vi "Main Traction Receipe Run.vi"(8 "error in (no error)":errorcluster, 11 "main ref":T1) -> (0 "error out":errorcluster)   [LabVIEW 2025]
uses:
  Traction Receipe Enum.ctl
  v06/controls/LAB-IQ UI Data.ctl
  Temperature/Temperature enum.ctl
  <vilib>/Utility/error.llb/Trim Whitespace One-Sided.vi
panel:
  out "error out 3":errorcluster
  out "error out 2":errorcluster
  in  "Enum - Menu":T2
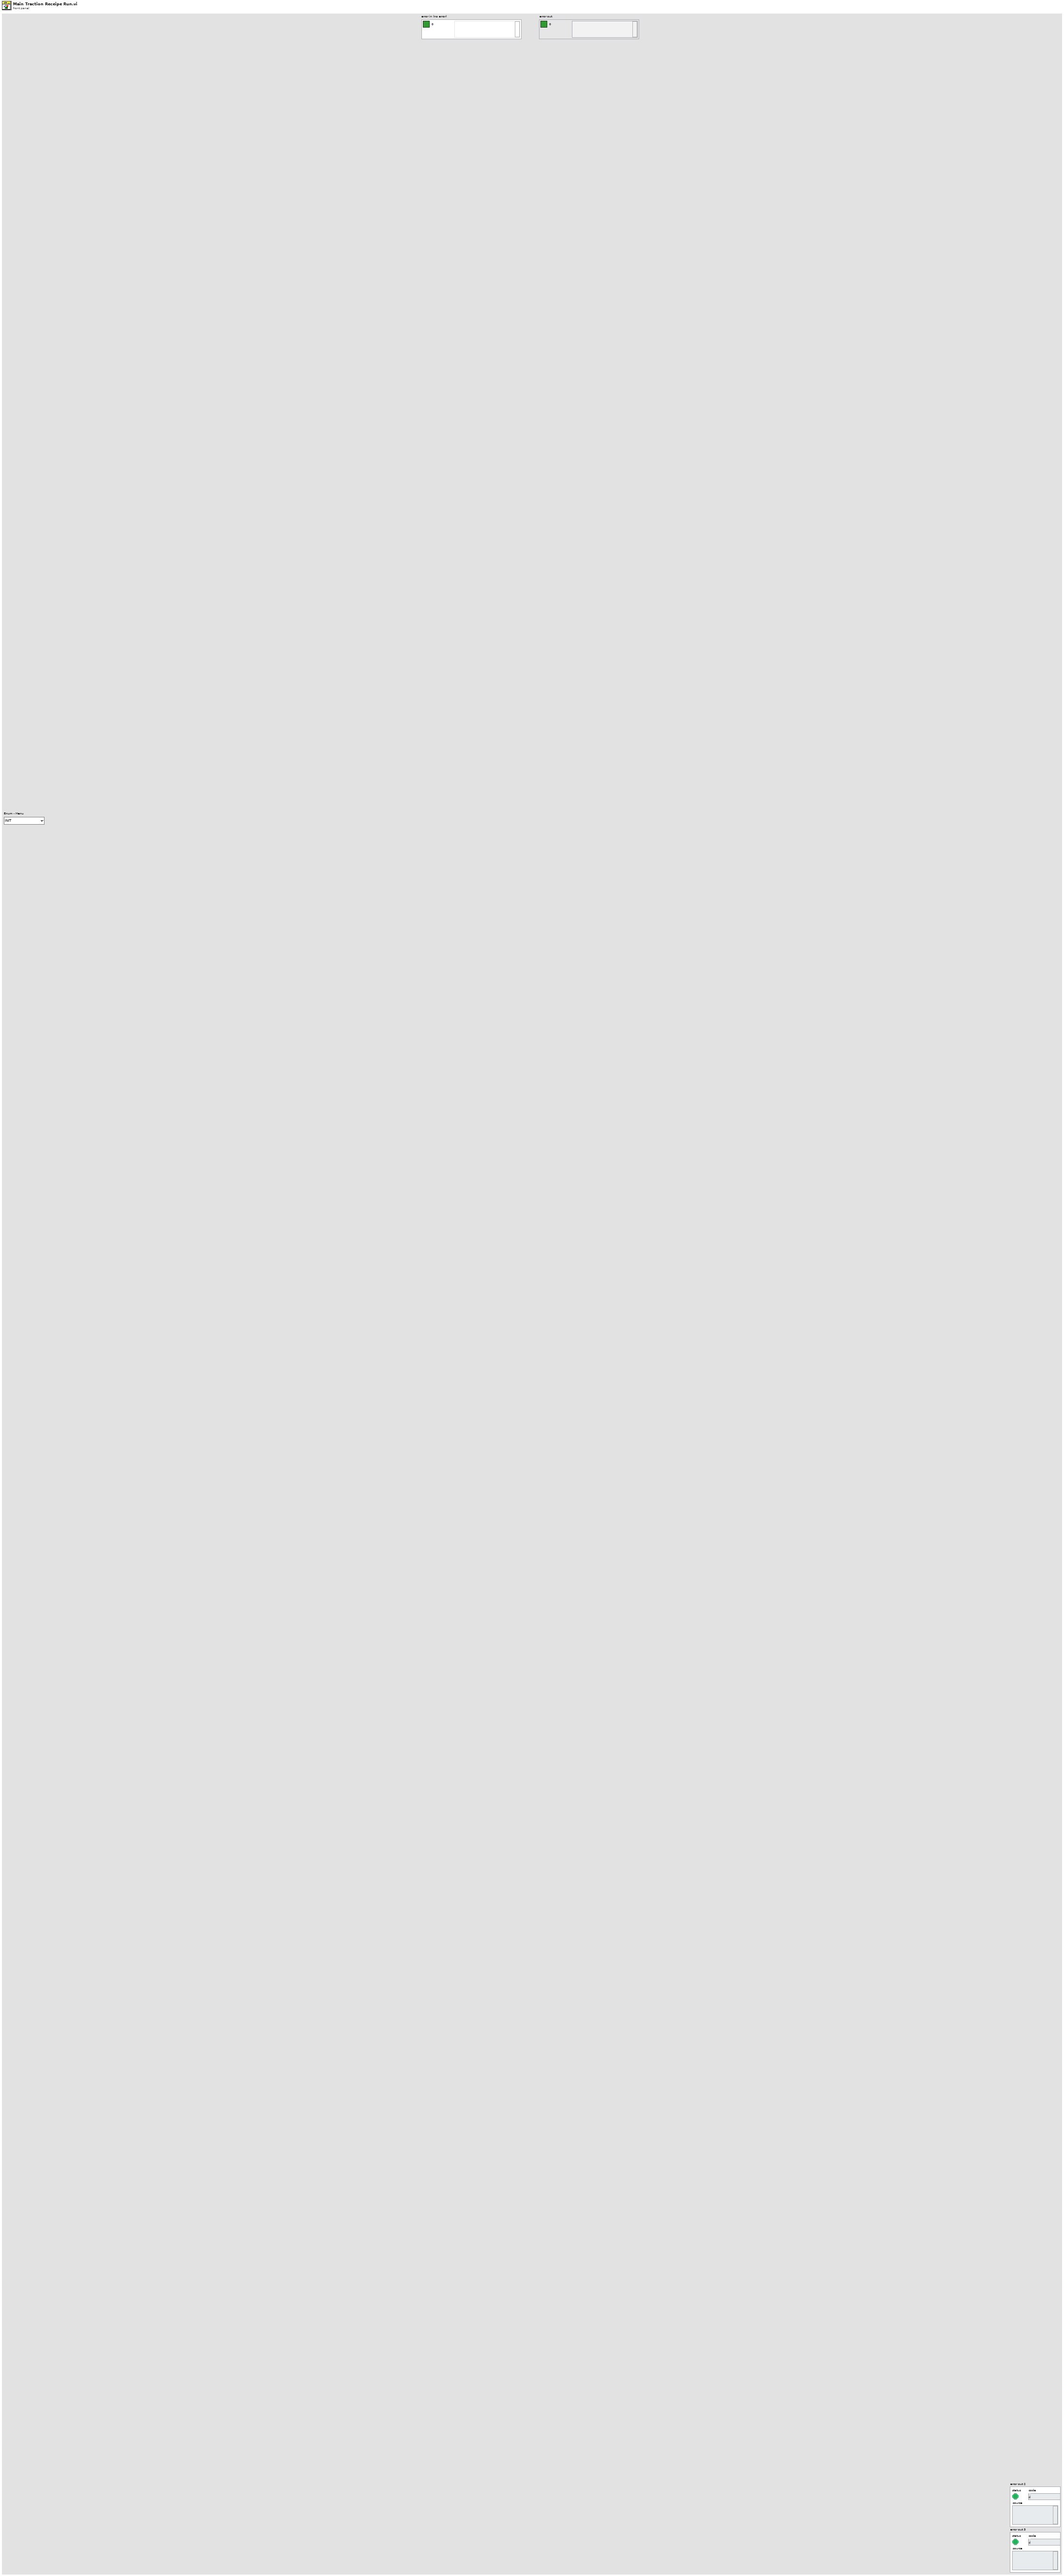
[diagram p1: front panel]
types:
  T1 = typedef "LAB-IQ UI Data.ctl" = cluster{"Main Home Screen":cluster{"GUI":refnum<vi>, "Platform Settings":refnum<vi>, "Configure":refnum<vi>, "Home":refnum<vi>, "EXIT":refnum<vi>, "service 2":refnum<vi>, "MainPage":refnum<vi>, "Analysis":refnum<vi>}, "Platform Settings":cluster{"mm/s  Surge":refnum<vi>, "Drive Error":refnum<vi>, "Disable Axis Jog Soft Limits":refnum<vi>, "mm/s  Sway":refnum<vi>, "Sway and Surge COM Status":refnum<vi>, "Heave COM Status":refnum<vi>, "Enable Platform":refnum<vi>, "Surge Forward Main":refnum<vi>, "Sway Right Main":refnum<vi>, "Sway Left Main":refnum<vi>, "Heave Down Main":refnum<vi>, "Heave Up main":refnum<vi>, "mm/s Heave":refnum<vi>, "mm/sec":refnum<vi>, "mm":refnum<vi>, "Surge Backward Main":refnum<vi>}, "Analysis Screen":cluster{"Analysis Home":refnum<vi>, "Surface Analysis":refnum<vi>, "Imaging":refnum<vi>, "Image Analysis":refnum<vi>, "Post Analysis":refnum<vi>}, "Config Screen":cluster{"Select Load Head":refnum<vi>, "Notes :":refnum<vi>, "FILE":refnum<vi>, "Sample ID :":refnum<vi>, "Operator ID :":refnum<vi>, "Operator Name :":refnum<vi>, "Auto":refnum<vi>}, "Motion Module":cluster{"zNL":refnum<vi>, "NL disp":refnum<vi>, "Rotary Tab":refnum<vi>, "Motion Direction:  3":refnum<vi>, "E.Velocity 2":refnum<vi>, "e.v/ssr 2":refnum<vi>, "Enter Fixed E.Velocity 2":refnum<vi>, "Enter Final SRR 2":refnum<vi>, "Enter initial SRR 2":refnum<vi>, "Enter Fixed SRR 2":refnum<vi>, "Enter the Final E.Velocity (m/s) 2":refnum<vi>, "Enter initial E.Velocity (m/s) 2":refnum<vi>, "Final Speed (RPM) 3":refnum<vi>, "Initial Speed (RPM) 2":refnum<vi>, "Enter the Final Velocity (m/s) 3":refnum<vi>, "Enter initial Velocity (m/s)  3":refnum<vi>, "Ramp Up 2":refnum<vi>, "TEST SELECTION":refnum<vi>, "SPEED SELECTION : ":refnum<vi>, "Angular Oscillation Set":refnum<vi>, "Traction":refnum<vi>, "Step Speed":refnum<vi>, "StepTable For Load-Speed":refnum<vi>, "StepTable For Speed":refnum<vi>, "Surge Forward MM":refnum<vi>, "Surge Backward MM":refnum<vi>, "M3 Image":refnum<vi>, "String 39":refnum<vi>, "Sway Left MM":refnum<vi>, "Sway Right MM":refnum<vi>, "Disable Axis Jog Soft Limits":refnum<vi>, "mm":refnum<vi>, "Heave Down MM":refnum<vi>, "Heave Up MM":refnum<vi>, "Wear Track Diameter (mm)":refnum<vi>, "Set WTD":refnum<vi>, "HomeScratch":refnum<vi>, "HomeRot":refnum<vi>, "PlaceModule":refnum<vi>, "Enter the Angle (Deg)":refnum<vi>, "Enter the Frequency (Hz)":refnum<vi>, "Motion Mode:":refnum<vi>, "LR Sway":refnum<vi>, "Rot Hor":refnum<vi>, "Scratch":refnum<vi>, "LR Cam":refnum<vi>, "MMBack":refnum<vi>, "MMNext":refnum<vi>, "Rot Ver":refnum<vi>, "Rotary Module Selection":refnum<vi>, "calculate rotary":refnum<vi>, "SPEED SELECTION : rotary":refnum<vi>, "Import 2":refnum<vi>, "Save 2":refnum<vi>, "File Path :  2":refnum<vi>, "String 45":refnum<vi>, "StepTable For Speed 3":refnum<vi>, "Enter the Speed(mm/sec)":refnum<vi>, "Enter the Speed(RPM)":refnum<vi>, "Enter Scratch Speed (mm/s):":refnum<vi>, "SwaySpeed Set":refnum<vi>, "Scartch Offset":refnum<vi>, "Motion type:":refnum<vi>, "HomeScratch 2":refnum<vi>, "Enter Scratch length (mm):":refnum<vi>, "Wear Track Diameter":refnum<vi>, "Rotary Speed Exced":refnum<vi>, "Scratch Mode":refnum<vi>, "No of Scratch":refnum<vi>}, "Environmental control":cluster{"Humidity  Status  3":refnum<vi>, "Low Temp  Status  2":refnum<vi>, "TK4 status 2":refnum<vi>, "Stage Temperature":refnum<vi>, "Sample Temperature":refnum<vi>, "Humidity (Amb)":refnum<vi>, "Clear List":refnum<vi>, "Add to list":refnum<vi>, "Wear":refnum<vi>, "Vibration":refnum<vi>, "Humidity (Chamber)":refnum<vi>, "Temperature (Chamber)":refnum<vi>, "ECR ":refnum<vi>, "Temperature (Amb)":refnum<vi>, "Microphone":refnum<vi>, "Acoustic Emission 3":refnum<vi>, "SNext":refnum<vi>, "APBack":refnum<vi>, "Enter the Temperature (°C):":refnum<vi>, "Enter the Stage \nTemperature (°C):":refnum<vi>, "Enter the Humidity (%Rh):":refnum<vi>, "Low Temp":refnum<vi>, "High Temp":refnum<vi>, "Humidity":refnum<vi>, "Sensors Picked":refnum<vi>}, "About Screen":cluster{"Password":refnum<vi>, "Home Service":refnum<vi>, "Advanced Setting":refnum<vi>, "About Tab":refnum<vi>, "ECR Port:":refnum<vi>, "Ramp Port:":refnum<vi>, "Installation/Replacement completed":refnum<vi>, "Loahead":refnum<vi>, "Heave and Surge COM Port:":refnum<vi>, "Sway COM Port:":refnum<vi>, "Temp Modbus:":refnum<vi>, "Humidity Port:":refnum<vi>, "Edit Gain Constants":refnum<vi>, "Save Gain Constants":refnum<vi>}, "Main Screen":cluster{"Main Screen Tab":refnum<vi>, "Angle and Frequency":refnum<vi>, "Stroke (mm)":refnum<vi>, "Angle (Deg)":refnum<vi>, "Main Speed Tab":refnum<vi>, "MTM MOTOR DISPLAY":refnum<vi>, "Disc Speed (m/sec)":refnum<vi>, "Ball Speed (m/sec)":refnum<vi>, "Disc Speed (RPM)":refnum<vi>, "Ball Speed (RPM)":refnum<vi>, "SPEED TAB":refnum<vi>, "Speed (m/sec)":refnum<vi>, "Set Speed (m/sec)":refnum<vi>, "Speed (RPM)":refnum<vi>, "Set Speed":refnum<vi>, "Time Tab":refnum<vi>, "Time ( HH:MM:SS ) 2":refnum<vi>, "Test Duration":refnum<vi>, "Test Duration 4":refnum<vi>, "TEST CYCLE":refnum<vi>, "TOTAL CYCLES":refnum<vi>, "Set Load (N)":refnum<vi>, "Temp Tabs":refnum<vi>, "Heater":refnum<vi>, "TK4 status":refnum<vi>, "ChamberTemp":refnum<vi>, "SetTmp":refnum<vi>, "Controller  Status":refnum<vi>, "ChamberTemp 2":refnum<vi>, "SetTmp 2":refnum<vi>, "Controller  Status 2":refnum<vi>, "ChamberTemp 3":refnum<vi>, "SetTmp 3":refnum<vi>, "Cooling":refnum<vi>, "Load Communication":refnum<vi>, "Ambient \nTemperature":refnum<vi>, "HumCOMStatus":refnum<vi>, "Ambient\n Humidity":refnum<vi>, "Freq (Hz)":refnum<vi>, "Load En":refnum<vi>, "NLt":refnum<vi>, "zNL 2":refnum<vi>, "Humidity On":refnum<vi>, "humidity disp":refnum<vi>, "Set Humidity":refnum<vi>, "NL disp 2":refnum<vi>, "Humidity On 2":refnum<vi>, "humidity disp 2":refnum<vi>, "Set Humidity 2":refnum<vi>, "NL disp 3":refnum<vi>, "AppLoadSeq scratch":refnum<vi>, "Stop Scratch":refnum<vi>, "ClrLog":refnum<vi>, "Trip Log":refnum<vi>, "STOP":refnum<vi>, "Start Test":refnum<vi>, "Test status":refnum<vi>, "AR Led":refnum<vi>, "Data":refnum<vi>, "Health":refnum<vi>, "Sway COM Status":refnum<vi>, "Heave COM Status":refnum<vi>, "Grp Tab":refnum<vi>, "Sub Graph":refnum<vi>, "SD (mm)":refnum<vi>, "Siliding distance Reset Graph":refnum<vi>, "SDGp":refnum<vi>, "Humidity Reset Graph":refnum<vi>, "HumrGp":refnum<vi>, "Acoustic Emission (mV)":refnum<vi>, "Aqucostic Reset Graph":refnum<vi>, "gACQUOS":refnum<vi>, "ECR RESET":refnum<vi>, "ECR":refnum<vi>, "Temperature Reset":refnum<vi>, "Acoustic Emission (mV) 2":refnum<vi>, "Aqucostic Reset Graph 2":refnum<vi>, "gACQUOS 2":refnum<vi>, "ECR RESET 2":refnum<vi>, "ECR 2":refnum<vi>, "Temperature Reset 2":refnum<vi>, "Temperature (deg c)":refnum<vi>, "Speed Reset Graph":refnum<vi>, "Speed Tab":refnum<vi>, "MTM DISC  SPEED":refnum<vi>, "MTM BALL SPEED":refnum<vi>, "speed mm/sec":refnum<vi>, "Hymidity":refnum<vi>, "Humidity Disable trip":refnum<vi>, "CoF Trip  2":refnum<vi>, "Depth Trip":refnum<vi>, "Weart Deapth":refnum<vi>, "Depth Reset Graph":refnum<vi>, "Weart":refnum<vi>, "Depthz":refnum<vi>, "Depth (µm)":refnum<vi>, "WearGp":refnum<vi>, "NL Trip 2":refnum<vi>, "Load pid":refnum<vi>, "Load Disable Trip":refnum<vi>, "Load Reset Graph":refnum<vi>, "NL Display 4":refnum<vi>, "Main Chart 3":refnum<vi>, "BACK":refnum<vi>, "Depth Trip 2":refnum<vi>, "COF TRIP ":refnum<vi>, "Friction Force (N)":refnum<vi>, "FF Reset Graph":refnum<vi>, "FF Disable Trip":refnum<vi>, "FF TRIP":refnum<vi>, "COF Disable Trip":refnum<vi>, "COF Reset Graph":refnum<vi>, "Start Test Temp":refnum<vi>, "zFF":refnum<vi>, "Friction Force (N) Graph":refnum<vi>, "Coefficient of Friction":refnum<vi>, "Scratch Start Test":refnum<vi>, "FF Tab":refnum<vi>, "Cyclic Friction Force (N)":refnum<vi>, "CZ FF":refnum<vi>, "Cyclic Friction Force (N) Graph":refnum<vi>, "Cyclic Coefficient of Friction":refnum<vi>, "Cyclic FF TRIP":refnum<vi>, "Cyclic FF Disable Trip":refnum<vi>, "cyclic COF Disable Trip":refnum<vi>, "cyclic COF TRIP":refnum<vi>, "cyclic COF Reset Graph":refnum<vi>, "Cyclic FF Reset Graph":refnum<vi>, "Test Trip":refnum<vi>, "Multi Scratch Pass":refnum<vi>, "Scratch Start Recording":refnum<vi>, "Coefficient of Friction 2":refnum<vi>, "Acoustic Emission":refnum<vi>, "Friction Force (N) 2":refnum<vi>, "Depth (Microns)":refnum<vi>, "Normal Load ( N )":refnum<vi>}, "Loading":cluster{"Indentation":refnum<vi>, "Reference Sample":refnum<vi>, "Load Cell Communication Slide":refnum<vi>, "com 3":refnum<vi>, "com":refnum<vi>, "DecaForce COM Status":refnum<vi>, "Update":refnum<vi>, "Clear 3":refnum<vi>, "seq":refnum<vi>, "Stribeck table":refnum<vi>, "Stribeck Table  For loading":refnum<vi>, "Loading Mode":refnum<vi>, "Enter the Final Load (N)":refnum<vi>, "Enter the CoF Trip":refnum<vi>, "Enter the Friction Force Trip":refnum<vi>, "Enter the Normal load Trip":refnum<vi>, "Enter the Load  (N)":refnum<vi>, "KiloForce":refnum<vi>, "DecaForce ":refnum<vi>, "MicroForce":refnum<vi>, "LHBack":refnum<vi>, "LHNext":refnum<vi>, "Enter the Loading Rate (N/min)":refnum<vi>, "Message":refnum<vi>, "Warning 2":refnum<vi>, "SSP 0.75":refnum<vi>, "SSP 0.5":refnum<vi>, "SSP 0.3":refnum<vi>, "Warning":refnum<vi>, "gui GIF":refnum<vi>, "Communication is established":refnum<vi>, "AppLoad 4":refnum<vi>, "Multipoint":refnum<vi>, "Load Selection":refnum<vi>}, "PID":cluster{"Ramp":refnum<vi>, "Vertical load (N)":refnum<vi>, "apply load":refnum<vi>, "apply load 2":refnum<vi>, "Enter ByPass Load":refnum<vi>, "Bypass Load":refnum<vi>, "gFF Rot":refnum<vi>}, "Config Parameters":cluster{"Tab Control 3":refnum<vi>, "Tab Control 19":refnum<vi>, "SAMPLES":refnum<vi>, "Re-initilaize":refnum<vi>, "Filter ON/OFF":refnum<vi>, "TracHomeSurgeOffsetCounts 10MM":refnum<vi>, "TracHomeSwayOffsetCounts 10MM":refnum<vi>, "Acoustic Emission:":refnum<vi>, "Apply Filter (FF)":refnum<vi>, "Filter% 2":refnum<vi>, "Apply Filter (Load)":refnum<vi>, "Filter% ":refnum<vi>, "Sway distance (mm)":refnum<vi>, "Surge distance (mm)":refnum<vi>, "DataSavingLoopDelay(ms)":refnum<vi>, "SAVE 2":refnum<vi>, "Enter Distance":refnum<vi>, "Sway Counts:":refnum<vi>, "Distance (mm): 3":refnum<vi>, "Surge Counts:":refnum<vi>, "Distance (mm): 2":refnum<vi>, "Distance (mm):":refnum<vi>, "Heave Counts:":refnum<vi>, "LRMHomeSurgeOffsetCounts":refnum<vi>, "LRMHomeSwayOffsetCounts":refnum<vi>, "TracHomeSurgeOffsetCounts 20MM":refnum<vi>, "TracHomeSwayOffsetCounts 20MM":refnum<vi>, "RotHomeSwayOffsetCounts":refnum<vi>, "RotHomeSurgeOffsetCounts":refnum<vi>, "Heave distance":refnum<vi>, "Zmm":refnum<vi>, "Heave Pulses/mm":refnum<vi>, "Surge Pulses/mm":refnum<vi>, "Sway Pulses/mm":refnum<vi>, "Heave Pitch":refnum<vi>, "Surge Pitch":refnum<vi>, "Sway Pitch":refnum<vi>, "Heave PPR":refnum<vi>, "Surge PPR":refnum<vi>, "Sway PPR":refnum<vi>, "Tab Control 5":refnum<vi>, "Tab Control 14":refnum<vi>, "Tab Control 26":refnum<vi>, "AE":refnum<vi>, "Heave Loop Delay":refnum<vi>, "Heave PID Speed":refnum<vi>, "Surge Jog Speed":refnum<vi>, "Heave Jog Speed":refnum<vi>, "Sway Loop Delay":refnum<vi>, "Sway PID Speed":refnum<vi>, "Sway Jog Speed":refnum<vi>, "DEPTH TRIP VALUE":refnum<vi>, "LOAD TRIP VALUE":refnum<vi>, "DEPTH TRIP   ENABLE":refnum<vi>, "LOAD TRIP  ENABLE":refnum<vi>, "CYCLIC FF TRIP VALUE":refnum<vi>, "FF TRIP VALUE":refnum<vi>, "CYCLIC CoF TRIP VALUE":refnum<vi>, "COF TRIP VALUE":refnum<vi>, "CYCLIC COF TRIP  ENABLE":refnum<vi>, "CYCLIC FF TRIP  ENABLE":refnum<vi>, "FF TRIP  ENABLE":refnum<vi>, "COF TRIP  ENABLE":refnum<vi>, "JOG TRIP LOAD VALUE (N)":refnum<vi>, "Rotary Vertical":refnum<vi>, "Traction":refnum<vi>, "Scratch":refnum<vi>, "LRM CAM":refnum<vi>, "Sway LRM":refnum<vi>, "Rotary Horizontal":refnum<vi>, "SURGE SPEED":refnum<vi>, "SURGE BACKWARD COUNT":refnum<vi>, "SURGE FORWARD COUNT":refnum<vi>, "Start Button":refnum<vi>}, "Loading Com Port":cluster{"ClearAll":refnum<vi>, "Mz(Nm)":refnum<vi>, "My(Nm)":refnum<vi>, "Mx(Nm)":refnum<vi>, "Save Dwell":refnum<vi>, "Acq Delay (ms)":refnum<vi>, "Burst Delay (ms)":refnum<vi>, "model":refnum<vi>, "SN":refnum<vi>, "FFx(N)":refnum<vi>, "Sensor IP":refnum<vi>, "Port":refnum<vi>, "FFy(N)":refnum<vi>, "Load(N)":refnum<vi>, "delete Handle":refnum<vi>, "Create Handle":refnum<vi>, "ft_data":refnum<vi>, "ft_range":refnum<vi>, "ft_data 2":refnum<vi>, "stop 6":refnum<vi>, "running_flag":refnum<vi>, "ft_udp_handle":refnum<vi>, "get-data-return":refnum<vi>, "get-range-return":refnum<vi>, "zero-return":refnum<vi>, "filter-return":refnum<vi>, "initial-return":refnum<vi>, "deleteHandle-result":refnum<vi>, "Load Cell Temp":refnum<vi>, "Load Cell":refnum<vi>, "ZeroAll":refnum<vi>, "FORCE (N)":refnum<vi>, "TORQUE (N-m)":refnum<vi>, "Load Cell Link":refnum<vi>}, "Heave AND Surge":cluster{"SURGE POSE":refnum<vi>, "error out Read":refnum<vi>, "HEAVE POSE":refnum<vi>, "State":refnum<vi>, "Homed":refnum<vi>, "Sequence ID":refnum<vi>, "error out Write":refnum<vi>, "faultCode":refnum<vi>, "Ack ID":refnum<vi>, "SPEED":refnum<vi>, "Distance":refnum<vi>, "Mode Command":refnum<vi>, "Heave and Surge Read":refnum<vi>, "Read Heave Temp":refnum<vi>, "Spare 15":refnum<vi>, "Spare 14":refnum<vi>, "Spare 13":refnum<vi>, "Spare 12":refnum<vi>, "Spare 11":refnum<vi>, "Spare 10":refnum<vi>, "Spare 9":refnum<vi>, "Spare 8":refnum<vi>, "Spare 7":refnum<vi>, "Spare 4":refnum<vi>, "Spare 3":refnum<vi>, "Spare 2":refnum<vi>, "Humidity":refnum<vi>, "Temp":refnum<vi>, "Node Id":refnum<vi>, "Spare 1":refnum<vi>, "SPARE 4":refnum<vi>, "SPARE 3":refnum<vi>, "SPARE 2":refnum<vi>, "SPARE 1":refnum<vi>, "fwMajor":refnum<vi>, "fwMinor":refnum<vi>, "Manual Write":refnum<vi>, "Heave and Surge Write":refnum<vi>, "SPARE 5":refnum<vi>, "Reserved ":refnum<vi>, "SPARE 8":refnum<vi>, "SPARE 6":refnum<vi>, "SPARE 7":refnum<vi>, "SPARE 17":refnum<vi>, "SPARE 16":refnum<vi>, "SPARE 15":refnum<vi>, "SPARE 14":refnum<vi>, "SPARE 13":refnum<vi>, "SPARE 12":refnum<vi>, "SPARE 11":refnum<vi>, "SPARE 10":refnum<vi>, "SPARE 9":refnum<vi>, "System UPTIME":refnum<vi>, "Missed Packets":refnum<vi>, "faultCode Surge Right":refnum<vi>, "faultCode Surge Left":refnum<vi>, "faultCode Heave":refnum<vi>, "UPLINK HEAVE":refnum<vi>, "DOWNLINK HEAVE":refnum<vi>}, "New PID LOGIC":cluster{"Fine Tune Zone":refnum<vi>, "PID SDelay":refnum<vi>, "Max_pos_limit":refnum<vi>, "Min_pos_limit":refnum<vi>, "i_limit":refnum<vi>, "pct_scale":refnum<vi>, "Deadband":refnum<vi>, "Kd":refnum<vi>, "Ki":refnum<vi>, "Kp":refnum<vi>, "Current Position":refnum<vi>, "Set Load":refnum<vi>, "Current Load":refnum<vi>, "Pulse delta":refnum<vi>, "Init Step":refnum<vi>, "Max Step Linit":refnum<vi>, "min_deadband_floor":refnum<vi>, "dynamic_spindle_noise_scalar":refnum<vi>, "min_finetune_floor":refnum<vi>, "filter_alpha":refnum<vi>, "PID":refnum<vi>}, "SWAY ":cluster{"fwMajor":refnum<vi>, "Homed":refnum<vi>, "Rotary POSE":refnum<vi>, "State":refnum<vi>, "SWAY POSE":refnum<vi>, "Ack ID":refnum<vi>, "faultCode":refnum<vi>, "Node Id":refnum<vi>, "fwMinor":refnum<vi>, "Spare 6":refnum<vi>, "Spare 5":refnum<vi>, "Spare 4":refnum<vi>, "Spare 3":refnum<vi>, "Spare 2":refnum<vi>, "Spare 1":refnum<vi>, "Spare 7":refnum<vi>, "SPARE  5":refnum<vi>, "error out Write  SWAY ":refnum<vi>, "error out Read SWAY ":refnum<vi>, "Manual Write SWAY ":refnum<vi>, "SWAY WRITE":refnum<vi>, "SPARE  4":refnum<vi>, "SPARE  3":refnum<vi>, "SPARE 2":refnum<vi>, "SPARE 1":refnum<vi>, "Spare 15":refnum<vi>, "Spare 14":refnum<vi>, "Spare 13":refnum<vi>, "Spare 12":refnum<vi>, "Spare 11":refnum<vi>, "Spare 9":refnum<vi>, "Spare 8":refnum<vi>, "SPEED":refnum<vi>, "Distance":refnum<vi>, "Mode Command":refnum<vi>, "Sequence ID":refnum<vi>, "SWAY READ":refnum<vi>, "Spare 10":refnum<vi>, "Read SWAY Temp":refnum<vi>, "faultCode Sway ":refnum<vi>, "Missed Packets":refnum<vi>, "System UPTIME sway":refnum<vi>, "SPARE 6":refnum<vi>, "SPARE 7":refnum<vi>, "SPARE 9":refnum<vi>, "SPARE 11":refnum<vi>, "SPARE 10":refnum<vi>, "SPARE 8":refnum<vi>, "SPARE 13":refnum<vi>, "SPARE 12":refnum<vi>, "SPARE 17":refnum<vi>, "SPARE 16":refnum<vi>, "SPARE 15":refnum<vi>, "SPARE 14":refnum<vi>, "Reserved":refnum<vi>, "faultCode Rotary":refnum<vi>, "UPLINK SWAY":refnum<vi>, "DOWNLINK SWAY":refnum<vi>}, "Analysis Screen":cluster{"Analysis Home":refnum<vi>, "Refresh 2":refnum<vi>, "MEAN 4":refnum<vi>, "SD 4":refnum<vi>, "VARIANCE 4":refnum<vi>, "MEAN  3":refnum<vi>, "SD  3":refnum<vi>, "VARIANCE  3":refnum<vi>, "MEAN 2":refnum<vi>, "SD  2":refnum<vi>, "VARIANCE 2":refnum<vi>, "MEAN":refnum<vi>, "SD":refnum<vi>, "VARIANCE":refnum<vi>, "File 4 Discription":refnum<vi>, "OPEN 4":refnum<vi>, "File Name 4":refnum<vi>, "OPEN 3":refnum<vi>, "File 3 Discription":refnum<vi>, "File Name 3":refnum<vi>, "Y-AXIS":refnum<vi>, "X-AXIS":refnum<vi>, "XY Graph":refnum<vi>, "File Name 2":refnum<vi>, "File Name 1":refnum<vi>, "OPEN 2":refnum<vi>, "OPEN 1":refnum<vi>, "File 1 Discription ":refnum<vi>, "File 2 Discription":refnum<vi>, "Export":refnum<vi>, "File Format":refnum<vi>}, "Traction":cluster{"faultCode Traction 2":refnum<vi>, "faultCode Traction 1":refnum<vi>, "Missed Packets":refnum<vi>, "System UPTIME Traction":refnum<vi>, "SPARE 17":refnum<vi>, "SPARE 16":refnum<vi>, "SPARE 15":refnum<vi>, "SPARE 14":refnum<vi>, "SPARE 13":refnum<vi>, "SPARE 12":refnum<vi>, "SPARE 11":refnum<vi>, "SPARE 10":refnum<vi>, "SPARE 9":refnum<vi>, "SPARE 8":refnum<vi>, "SPARE 7":refnum<vi>, "SPARE 6":refnum<vi>, "Reserved":refnum<vi>, "SPARE  5":refnum<vi>, "Manual Write TRACTION":refnum<vi>, "TRACTION WRITE":refnum<vi>, "SPARE  4":refnum<vi>, "SPARE  3":refnum<vi>, "SPARE 2":refnum<vi>, "SPARE 1":refnum<vi>, "Spare 7":refnum<vi>, "Spare 6":refnum<vi>, "Spare 5":refnum<vi>, "Spare 4":refnum<vi>, "Spare 2":refnum<vi>, "Spare 1":refnum<vi>, "Node Id":refnum<vi>, "Read TRACTION Temp":refnum<vi>, "fwMinor":refnum<vi>, "fwMajor":refnum<vi>, "faultCode":refnum<vi>, "TRACTION POSE":refnum<vi>, "TRACTION POSE 2":refnum<vi>, "Homed":refnum<vi>, "State":refnum<vi>, "Ack ID":refnum<vi>, "SPEED":refnum<vi>, "Distance":refnum<vi>, "Mode Command":refnum<vi>, "Sequence ID":refnum<vi>, "error out Read TRACTION":refnum<vi>, "error out Write  TRACTION":refnum<vi>, "TRACTION READ":refnum<vi>, "Spare 3":refnum<vi>, "Downlink traction":refnum<vi>, "Uplink Traction":refnum<vi>}, "Traction reciepe":cluster{"SRR Sweep Range (%) Stribeck":refnum<vi>, "Traction Receipe":refnum<vi>, "Total Execution Time":refnum<vi>, "Total Steps":refnum<vi>, "Duration / Step (s)  Stribeck":refnum<vi>, "STRIBECK Fixed SRR List (%)":refnum<vi>, "Duration / Step (s) Traction":refnum<vi>, "SRR Sweep Range (%) traction":refnum<vi>, "Rolling Speed (mm/s)":refnum<vi>, "Temperature Stages (°C)":refnum<vi>, "Ball Load (N)":refnum<vi>, "Lubricant Name":refnum<vi>, "Profile File Name":refnum<vi>, "SET entrainment Velocity":refnum<vi>, "Test Array Size":refnum<vi>, "SRR INDEX [ STRIBECK]":refnum<vi>, "Stribeck Size":refnum<vi>, "SET SRR":refnum<vi>, "ELAPSED TIMER ":refnum<vi>, "BALL SET RPM":refnum<vi>, "DISC SET RPM":refnum<vi>, "SET LOAD":refnum<vi>, "TEMPERATURE READ":refnum<vi>, "SET TEMPERATURE":refnum<vi>, "Traction Size":refnum<vi>, "DISC SPEED (rpm)":refnum<vi>, "BALL SPEED (rpm)":refnum<vi>, "BALL WEAR TRACK":refnum<vi>, "DISC WEARTRACK":refnum<vi>, "SRR INDEX [ TRACTION]":refnum<vi>, "Start Index Type":refnum<vi>, "Enum - Menu":refnum<vi>, "Ball (mm/sec)":refnum<vi>, "Disc (mm/sec)":refnum<vi>, "Traction Receipe Update Details":refnum<vi>}, "Traction Control":cluster{"HomeTraction":refnum<vi>, "Demo Mode Display":refnum<vi>, "Traction Message":refnum<vi>, "Traction Step Update Details":refnum<vi>, "Main Tab sequence for selection":refnum<vi>, "Ramp Tab":refnum<vi>, "e.v/ssr":refnum<vi>, "Enter Fixed E.Velocity":refnum<vi>, "Enter Final SRR":refnum<vi>, "Enter initial SRR":refnum<vi>, "Enter Fixed SRR":refnum<vi>, "Enter the Final E.Velocity (m/s)":refnum<vi>, "Enter initial E.Velocity (m/s)":refnum<vi>, "Ball WTD":refnum<vi>, "E.Velocity":refnum<vi>, "Enter the Final Velocity (m/s)":refnum<vi>, "Enter initial Velocity (m/s)":refnum<vi>, "Ramp Up   Disc":refnum<vi>, "Initial DiscSpeed (RPM)":refnum<vi>, "Final Speed (RPM) Ball":refnum<vi>, "Final Speed (RPM)":refnum<vi>, "Initial Speed (RPM) Ball":refnum<vi>, "Enter the Final Velocity (m/s) Ball":refnum<vi>, "Enter initial Velocity (m/s) Ball":refnum<vi>, "Ramp Up":refnum<vi>, "ExceedBallSpeed step":refnum<vi>, "ExceedDiscSpeed":refnum<vi>, "BallSpeed Exceed Indication":refnum<vi>, "Apply":refnum<vi>, "SPEED SELECTION : MTM":refnum<vi>, "SPEED SELECTION : MTM 2":refnum<vi>, "TEST SELECTION (MTM)":refnum<vi>, "MTM Test Selection":refnum<vi>, "File Path Tab":refnum<vi>, "File Path String":refnum<vi>, "Save":refnum<vi>, "Save  2":refnum<vi>, "Import ":refnum<vi>, "File Path :":refnum<vi>, "Step Sequence Indication Tab":refnum<vi>, "Step Sequence Indication":refnum<vi>, "Calculate Step":refnum<vi>, "StepTable":refnum<vi>, "ExceedDiscSpeed  Cinstant Speed":refnum<vi>, "ExceedBallSpeed Constant":refnum<vi>, "TEST SELECTION (MTM) 2":refnum<vi>, "SPEED SELECTION : MTM 3":refnum<vi>, "MTM Test Selection 2":refnum<vi>, "Enter the Speed (m/sec): ":refnum<vi>, "Enter the Speed (m/sec):  2":refnum<vi>, "Enter the Speed (RPM):":refnum<vi>, "Lower Spped ":refnum<vi>, "Upper":refnum<vi>, "Enter the Speed (RPM):Ball":refnum<vi>, "Disc Motion Direction: ":refnum<vi>, "Ball Motion Direction :":refnum<vi>, "Motion Mode: ":refnum<vi>, "Wear Track Diameter (mm) ":refnum<vi>, "Disc Speed Indicator":refnum<vi>, "ExceedBallSpeed":refnum<vi>}, "Acquostic":cluster{"Last Config Rejected ":refnum<vi>, "rx command count":refnum<vi>, "Current Filter Id":refnum<vi>, "Isolated Gain":refnum<vi>, "DAQ Status":refnum<vi>, "error out":refnum<vi>, "error in (no error)":refnum<vi>, "Uplink Packet":refnum<vi>, "data out":refnum<vi>, "Downlink Packet":refnum<vi>, "Gains":refnum<vi>, "Manual Write Acquostic":refnum<vi>, "Acoustic Graphs":refnum<vi>}, "ABOUT":cluster{"version":refnum<vi>, "Operating System":refnum<vi>, "Version":refnum<vi>, "Workorder":refnum<vi>, "Runtime":refnum<vi>, "Instrument Serial":refnum<vi>, "Firmware Version":refnum<vi>, "Info":refnum<vi>}, "Temperature Port":cluster{"Temperature":refnum<vi>, "error out Temperature":refnum<vi>, "READ TEMPERATURE":refnum<vi>}}
  T2 = typedef "Traction Receipe Enum.ctl" = enum16{"INIT", "START", "TRACTION", "STRIBECK", "MAIN INDEX INCREMENT", "TEMPERATURE SET", "TEMPERATURE REACH", "CHURNING START", "CHURNING STOP", "LOAD", "LOAD REACHED", "SRR SET", "SRR WAIT", "SRR INCREMENT", "SPEED SET", "SPEED WAIT", "SPEED INCREMENT", "UNLOAD", "CLOSE"}
  T3 = typedef "Temperature enum.ctl" = enum16{"Init", "read", "write", "close", "error_init"}
  T4 = enum8{"Enabled", "Disabled", "Disabled and Grayed Out"}
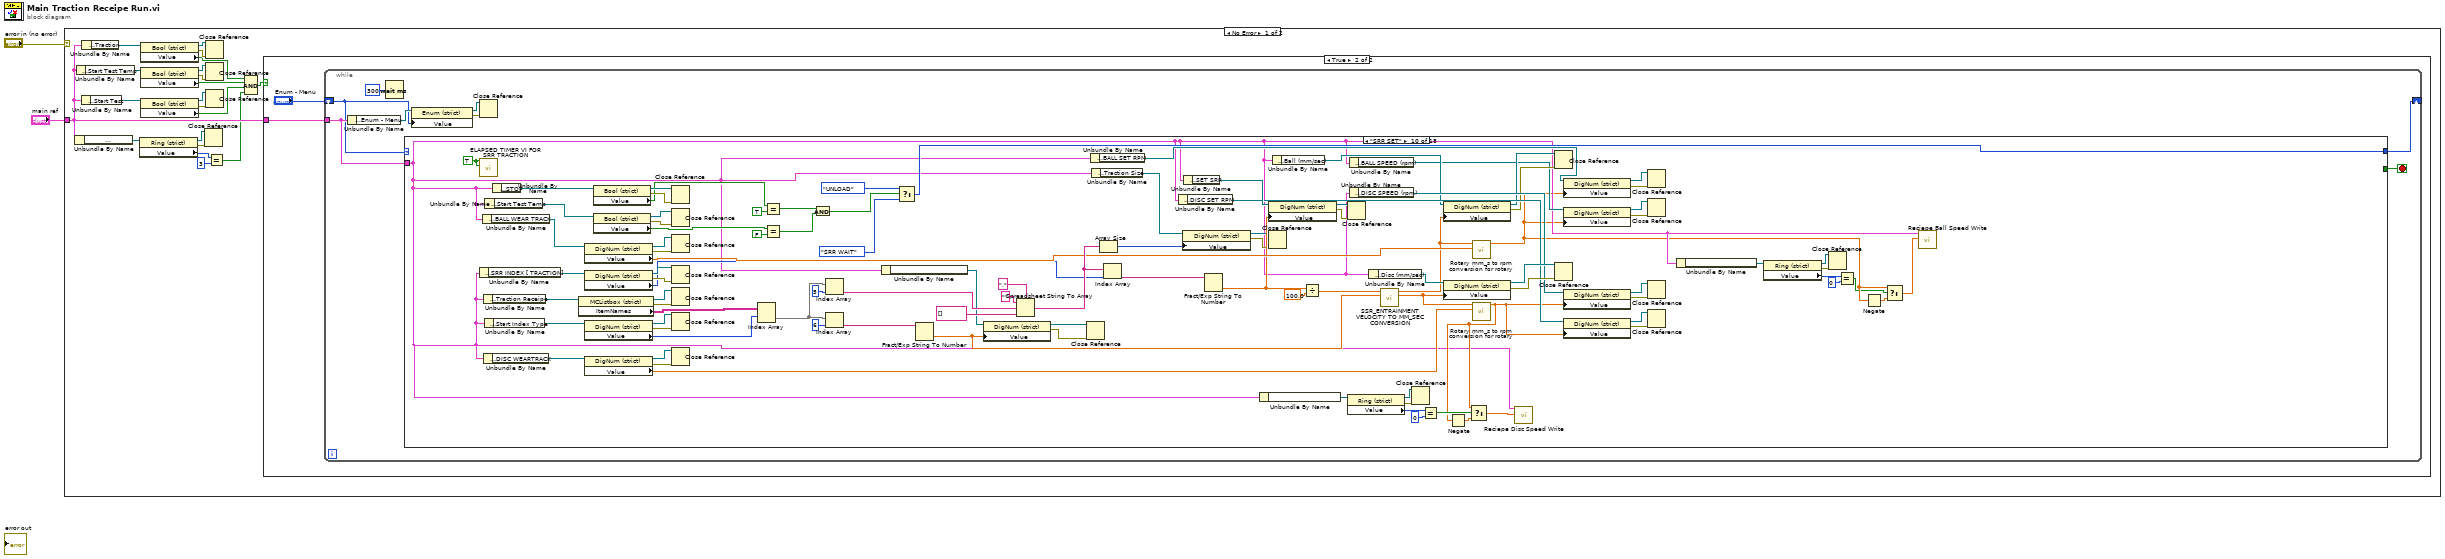
[diagram p0: block diagram]
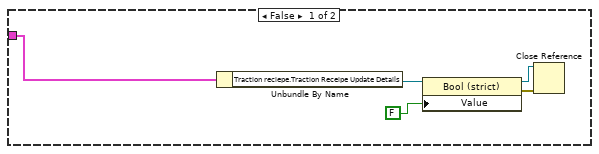
[diagram p2: hidden frame]
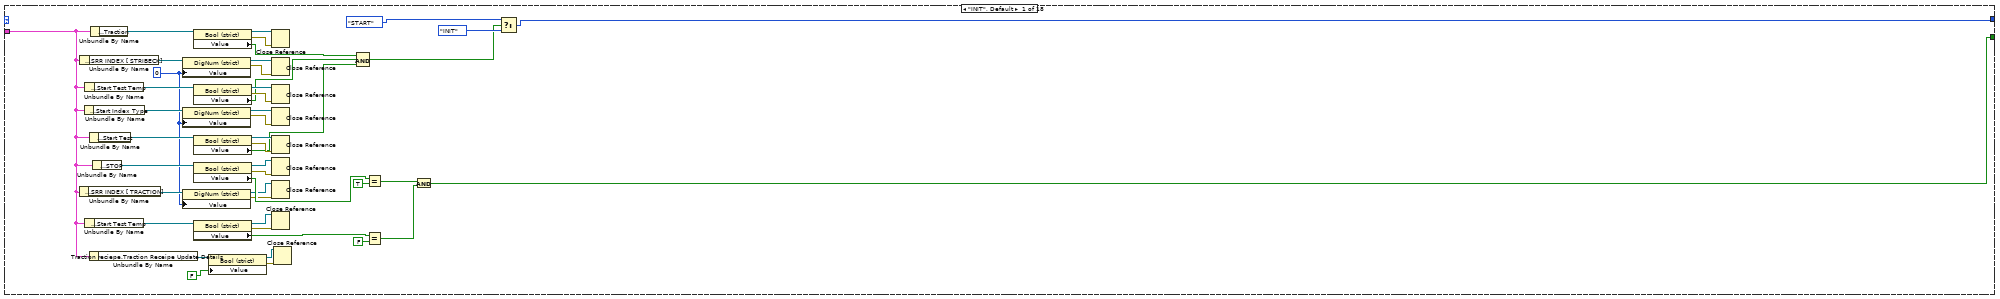
[diagram p3: hidden frame]
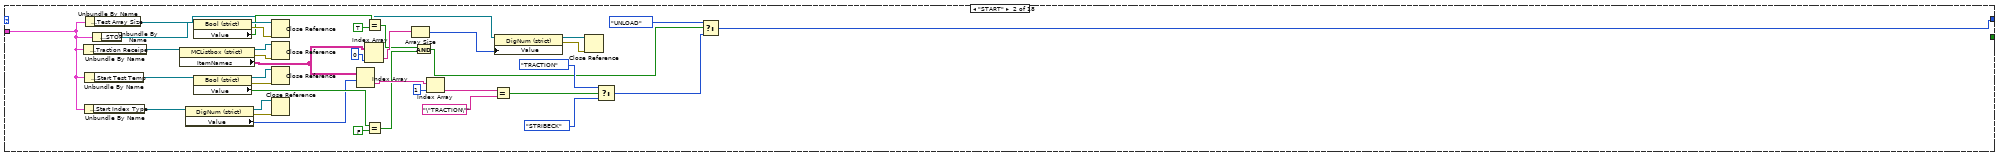
[diagram p4: hidden frame]
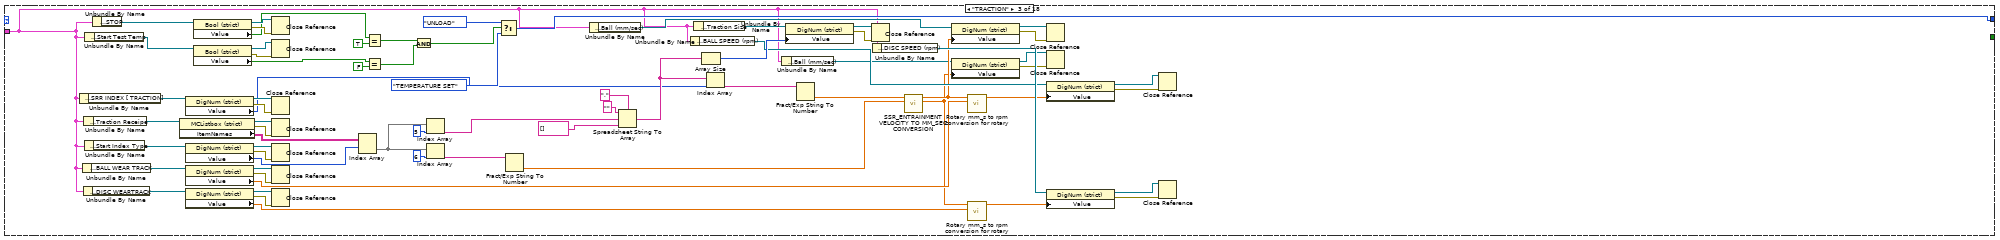
[diagram p5: hidden frame]
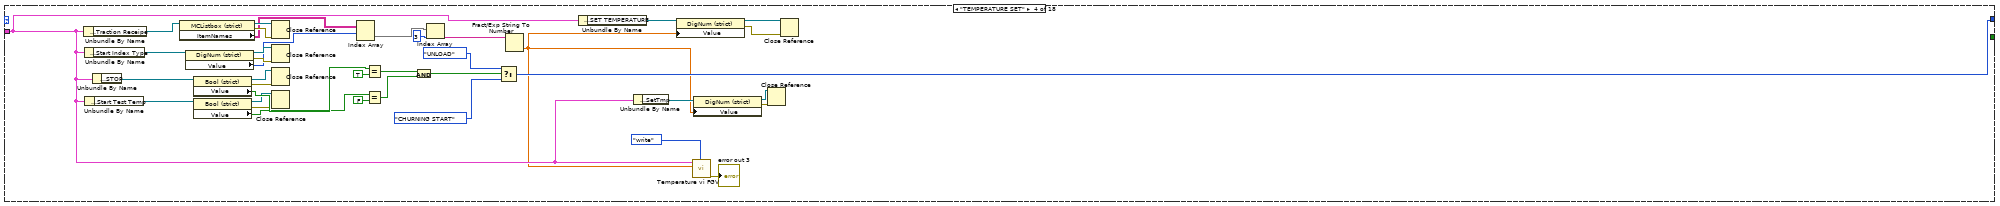
[diagram p6: hidden frame]
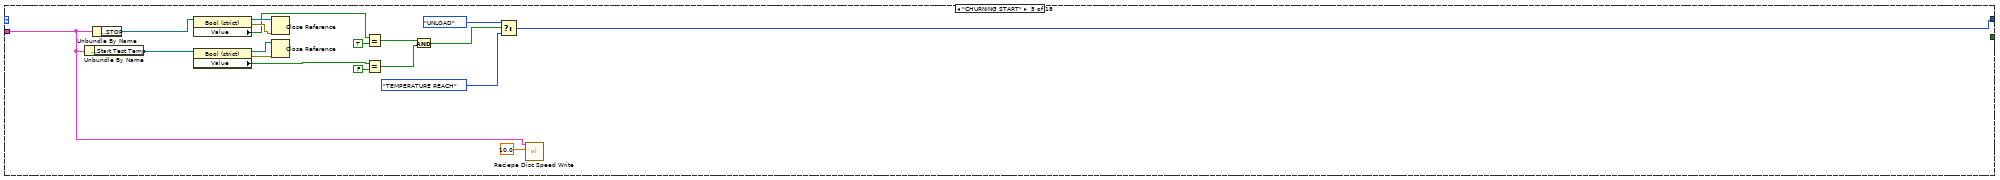
[diagram p7: hidden frame]
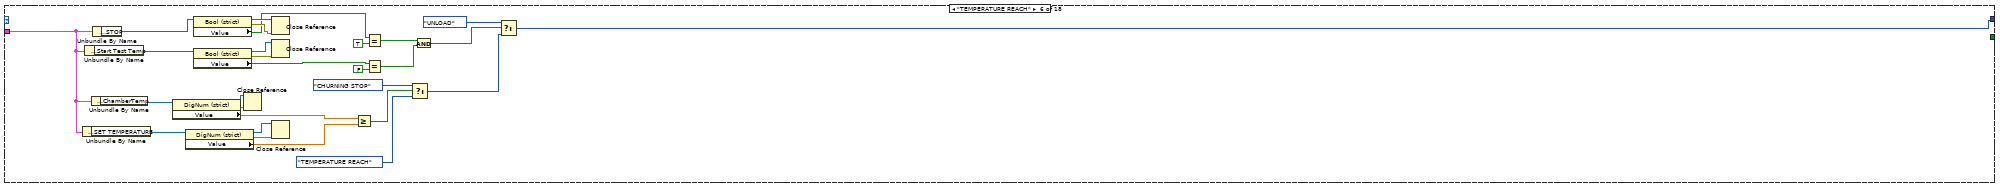
[diagram p8: hidden frame]
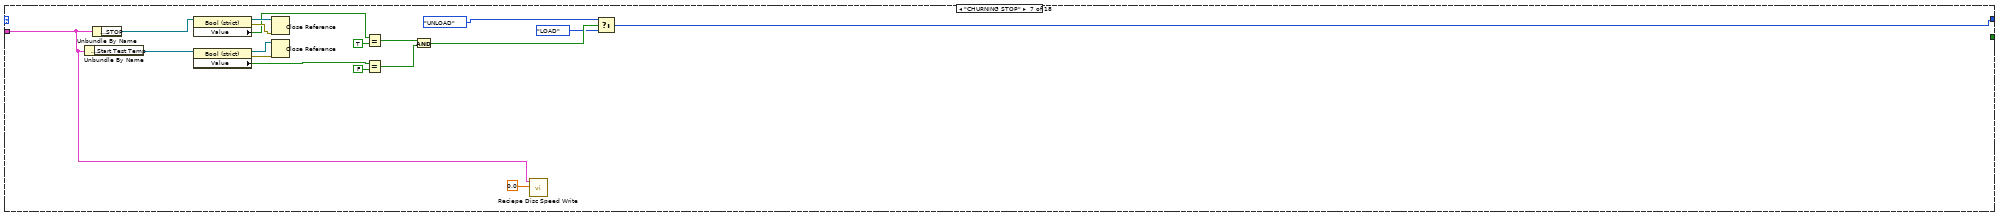
[diagram p9: hidden frame]
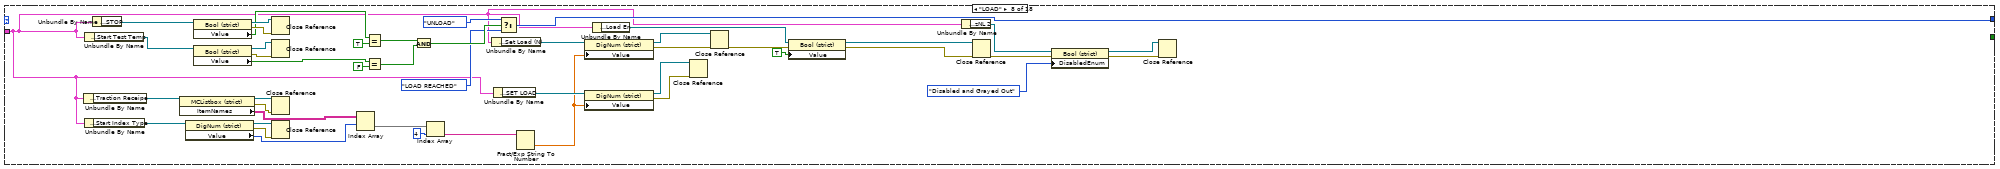
[diagram p10: hidden frame]
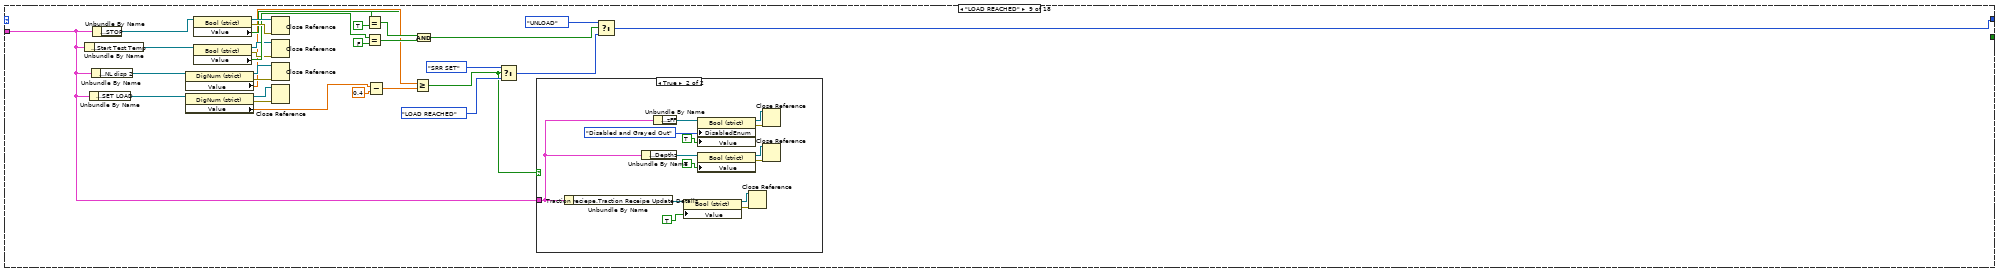
[diagram p11: hidden frame]
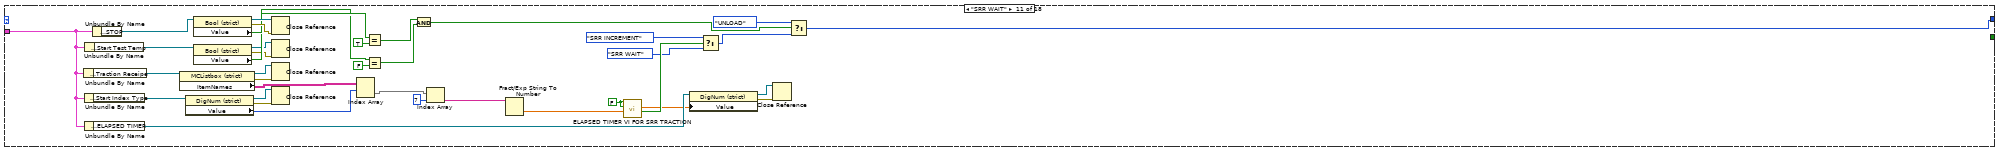
[diagram p13: hidden frame]
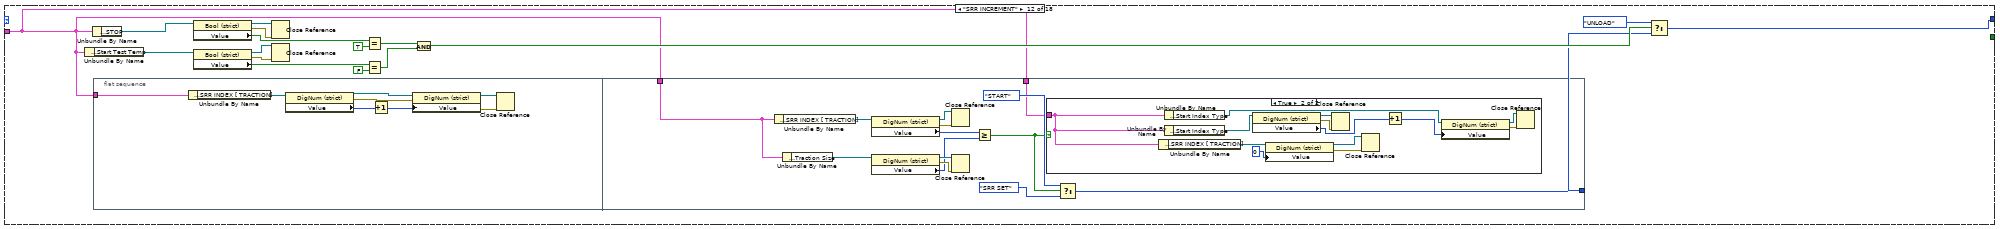
[diagram p14: hidden frame]
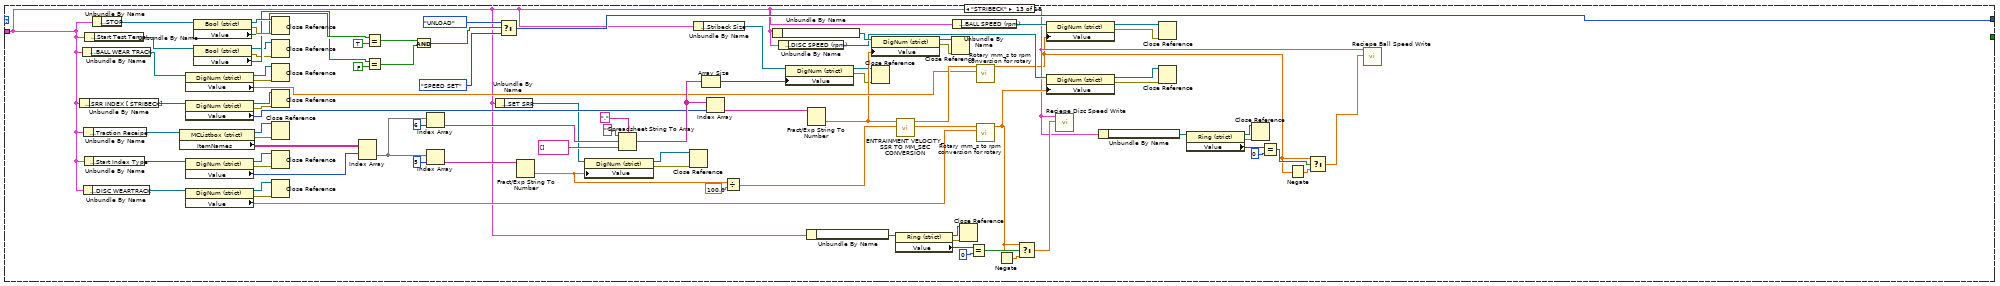
[diagram p16: hidden frame]
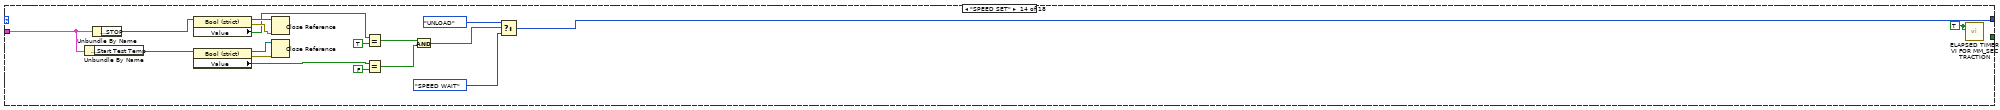
[diagram p17: hidden frame]
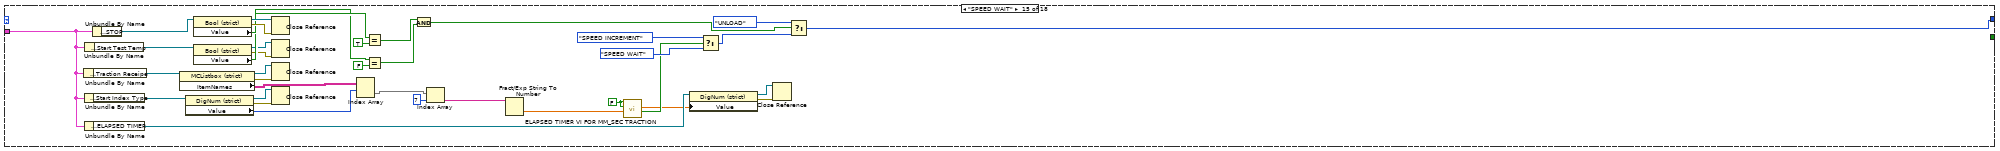
[diagram p18: hidden frame]
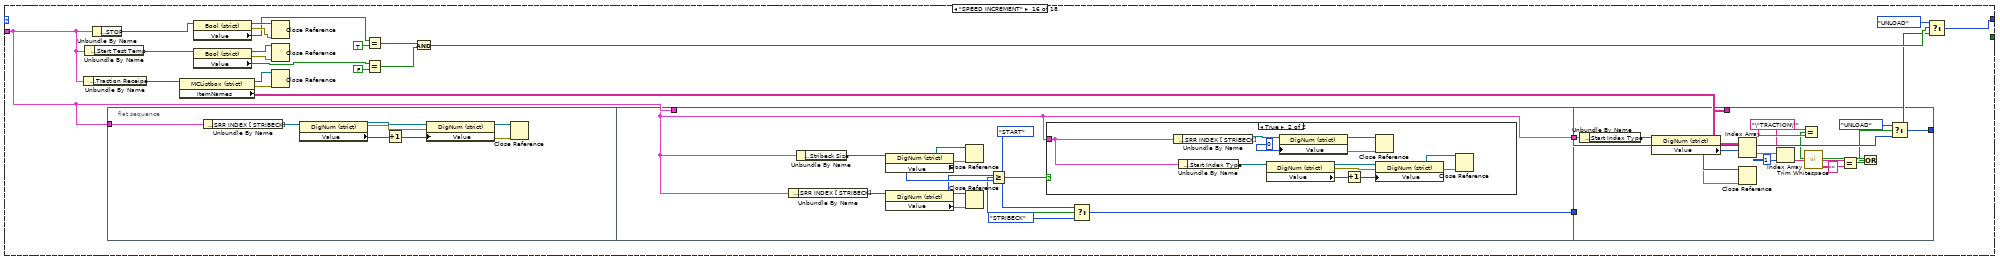
[diagram p19: hidden frame]
diagram:
  n1 = case shown="No Error" "error in (no error)" {
    tunnel: "main ref" -> [w6 _]
    frame No Error {
      n2 = Unbundle By Name(w6) -> ("Traction Control.Motion Mode:"=w8:refnum<vi>)
      n3 = Unbundle By Name(w6) -> ("Main Screen.Start Test Temp"=w21:refnum<vi>)
      n4 = Unbundle By Name(w6) -> ("Main Screen.Start Test"=w18:refnum<vi>)
      n5 = Unbundle By Name(w6) -> ("Motion Module.Traction"=w13:refnum<vi>)
      n6 = property class="Ring (strict)"(reference=w8) -> (reference out=w9:refnum<vi>, error out=w7:errorcluster, "Value"=w5:u16)  [unwired: 1 in]
      n7 = property class="Bool (strict)"(reference=w13) -> (reference out=w12:refnum<vi>, error out=w14:errorcluster, "Value"=w11:bool)  [unwired: 1 in]
      n8 = property class="Bool (strict)"(reference=w21) -> (reference out=w22:refnum<vi>, error out=w20:errorcluster, "Value"=w16:bool)  [unwired: 1 in]
      n9 = property class="Bool (strict)"(reference=w18) -> (reference out=w17:refnum<vi>, error out=w19:errorcluster, "Value"=w15:bool)  [unwired: 1 in]
      n10 = Close Reference(reference=w9, error in (no error)=w7) -> ()  [unwired: 1 out]
      n11 = Close Reference(reference=w12, error in (no error)=w14) -> ()  [unwired: 1 out]
      n12 = Close Reference(reference=w22, error in (no error)=w20) -> ()  [unwired: 1 out]
      n13 = Close Reference(reference=w17, error in (no error)=w19) -> ()  [unwired: 1 out]
      n14 = Equal?(x=w5, y=u16 3) -> (x = y?=w3:bool)
      n15 = Compound Arithmetic op=AND(w11, w16, w15, w3) -> (w10:bool)
      n16 = case shown="True" w10 {
        tunnel: w6 -> [w25 w28]
        frame False {
          n17 = Unbundle By Name(w25) -> ("Traction reciepe.Traction Receipe Update Details"=w26:refnum<vi>)
          n18 = property class="Bool (strict)"(reference=w26, "Value"=FALSE) -> (reference out=w24:refnum<vi>, error out=w27:errorcluster)  [unwired: 1 in]
          n19 = Close Reference(reference=w24, error in (no error)=w27) -> ()  [unwired: 1 out]
        }
        frame True {
          n20 = while {
            shift-right: [w37] -> _
            shift-left: "Enum - Menu" -> [w30]
            tunnel: w28 -> [w32]
            stop <- w36 stop-if-true
            n21 = Unbundle By Name(w32) -> ("Traction reciepe.Enum - Menu"=w33:refnum<vi>)
            n22 = Wait (ms)(milliseconds to wait=u32 300) -> ()  [unwired: 1 out]
            n23 = case shown="\"SRR SET\"" w30 {
              tunnel: [w79 w92 w162 w208 w228 w253 w274 w316 w347 w452 w492 w517 w627 w655 w686 w716 w810 Traction_Receipe_Enum."INIT" ("Enum - Menu")] -> w37
              tunnel: [w57 _ _ _ _ _ _ _ _ _ _ _ _ _ _ _ _ TRUE] -> w36
              tunnel: w32 -> [w38 w83 w121 w192 w226 w245 w272 w291 w336 w383 w480 w516 w570 w657 w674 w710 w784 w832]
              frame "INIT", Default {
                w43 = 0 ("Value")
                n24 = Unbundle By Name(w38) -> ("Traction reciepe.SRR INDEX [ TRACTION]"=w48:refnum<vi>)
                n25 = Unbundle By Name(w38) -> ("Traction reciepe.SRR INDEX [ STRIBECK]"=w51:refnum<vi>)
                n26 = Unbundle By Name(w38) -> ("Traction reciepe.Start Index Type"=w45:refnum<vi>)
                n27 = Unbundle By Name(w38) -> ("Main Screen.Start Test Temp"=w77:refnum<vi>)
                n28 = Unbundle By Name(w38) -> ("Main Screen.Start Test Temp"=w64:refnum<vi>)
                n29 = Unbundle By Name(w38) -> ("Traction reciepe.Traction Receipe Update Details"=w41:refnum<vi>)
                n30 = Unbundle By Name(w38) -> ("Main Screen.Start Test"=w74:refnum<vi>)
                n31 = Unbundle By Name(w38) -> ("Motion Module.Traction"=w55:refnum<vi>)
                n32 = Unbundle By Name(w38) -> ("Main Screen.STOP"=w67:refnum<vi>)
                n33 = property class="DigNum (strict)"(reference=w51, "Value"=w43) -> (reference out=w50:refnum<vi>, error out=w52:errorcluster)  [unwired: 1 in]
                n34 = property class="DigNum (strict)"(reference=w45, "Value"=w43) -> (reference out=w44:refnum<vi>, error out=w46:errorcluster)  [unwired: 1 in]
                n35 = property class="DigNum (strict)"(reference=w48, "Value"=w43) -> (reference out=w49:refnum<vi>, error out=w47:errorcluster)  [unwired: 1 in]
                n36 = property class="Bool (strict)"(reference=w55) -> (reference out=w54:refnum<vi>, error out=w56:errorcluster, "Value"=w53:bool)  [unwired: 1 in]
                n37 = property class="Bool (strict)"(reference=w77) -> (reference out=w78:refnum<vi>, error out=w76:errorcluster, "Value"=w72:bool)  [unwired: 1 in]
                n38 = property class="Bool (strict)"(reference=w74) -> (reference out=w73:refnum<vi>, error out=w75:errorcluster, "Value"=w71:bool)  [unwired: 1 in]
                n39 = property class="Bool (strict)"(reference=w67) -> (reference out=w69:refnum<vi>, error out=w68:errorcluster, "Value"=w66:bool)  [unwired: 1 in]
                n40 = property class="Bool (strict)"(reference=w64) -> (reference out=w62:refnum<vi>, error out=w63:errorcluster, "Value"=w65:bool)  [unwired: 1 in]
                n41 = property class="Bool (strict)"(reference=w41, "Value"=FALSE) -> (reference out=w40:refnum<vi>, error out=w42:errorcluster)  [unwired: 1 in]
                n42 = Close Reference(reference=w54, error in (no error)=w56) -> ()  [unwired: 1 out]
                n43 = Close Reference(reference=w50, error in (no error)=w52) -> ()  [unwired: 1 out]
                n44 = Close Reference(reference=w78, error in (no error)=w76) -> ()  [unwired: 1 out]
                n45 = Close Reference(reference=w44, error in (no error)=w46) -> ()  [unwired: 1 out]
                n46 = Close Reference(reference=w73, error in (no error)=w75) -> ()  [unwired: 1 out]
                n47 = Close Reference(reference=w69, error in (no error)=w68) -> ()  [unwired: 1 out]
                n48 = Close Reference(reference=w49, error in (no error)=w47) -> ()  [unwired: 1 out]
                n49 = Close Reference(reference=w62, error in (no error)=w63) -> ()  [unwired: 1 out]
                n50 = Close Reference(reference=w40, error in (no error)=w42) -> ()  [unwired: 1 out]
                n51 = Compound Arithmetic op=AND(w53, w72, w71) -> (w70:bool)
                n52 = Equal?(x=w66, y=TRUE) -> (x = y?=w61:bool)
                n53 = Equal?(x=w65, y=FALSE) -> (x = y?=w60:bool)
                n54 = And(x=w61, y=w60) -> (x .and. y?=w57:bool)
                n55 = Select(t=Traction_Receipe_Enum."START" ("Enum - Menu"), s=w70, f=Traction_Receipe_Enum."INIT" ("Enum - Menu")) -> (s? t:f=w79:T2)
              }
              frame "START" {
                n56 = Unbundle By Name(w83) -> ("Traction reciepe.Traction Receipe"=w110:refnum<vi>)
                n57 = Unbundle By Name(w83) -> ("Traction reciepe.Start Index Type"=w85:refnum<vi>)
                n58 = Unbundle By Name(w83) -> ("Main Screen.Start Test Temp"=w101:refnum<vi>)
                n59 = Unbundle By Name(w83) -> ("Traction reciepe.Test Array Size"=w89:refnum<vi>)
                n60 = Unbundle By Name(w83) -> ("Main Screen.STOP"=w104:refnum<vi>)
                n61 = property class="MCListbox (strict)"(reference=w110) -> (reference out=w108:refnum<vi>, error out=w109:errorcluster, "ItemNames"=w107:string[][])  [unwired: 1 in]
                n62 = property class="DigNum (strict)"(reference=w85) -> (reference out=w84:refnum<vi>, error out=w86:errorcluster, "Value"=w82:i32)  [unwired: 1 in]
                n63 = property class="Bool (strict)"(reference=w104) -> (reference out=w106:refnum<vi>, error out=w105:errorcluster, "Value"=w103:bool)  [unwired: 1 in]
                n64 = property class="Bool (strict)"(reference=w101) -> (reference out=w99:refnum<vi>, error out=w100:errorcluster, "Value"=w102:bool)  [unwired: 1 in]
                n65 = Close Reference(reference=w106, error in (no error)=w105) -> ()  [unwired: 1 out]
                n66 = Close Reference(reference=w108, error in (no error)=w109) -> ()  [unwired: 1 out]
                n67 = Close Reference(reference=w99, error in (no error)=w100) -> ()  [unwired: 1 out]
                n68 = Close Reference(reference=w84, error in (no error)=w86) -> ()  [unwired: 1 out]
                n69 = Index Array(array=w107, index (row)=w82) -> (element=w116:string[])  [unwired: 1 in]
                n70 = Index Array(array=w107, index (col)=0 ("index (row)")) -> (element=w112:string[])  [unwired: 1 in]
                n71 = Equal?(x=w103, y=TRUE) -> (x = y?=w98:bool)
                n72 = Equal?(x=w102, y=FALSE) -> (x = y?=w97:bool)
                n73 = Array Size(array=w112) -> (size(s)=w87:i32)
                n74 = And(x=w98, y=w97) -> (x .and. y?=w94:bool)
                n75 = Index Array(array=w116, index=1) -> (element=w118:string)
                n76 = Equal?(x=w118, y="\"TRACTION\"") -> (x = y?=w113:bool)
                n77 = property class="DigNum (strict)"(reference=w89, "Value"=w87) -> (reference out=w88:refnum<vi>, error out=w90:errorcluster)  [unwired: 1 in]
                n78 = Close Reference(reference=w88, error in (no error)=w90) -> ()  [unwired: 1 out]
                n79 = Select(t=Traction_Receipe_Enum."TRACTION" ("Enum - Menu"), s=w113, f=Traction_Receipe_Enum."STRIBECK" ("Enum - Menu")) -> (s? t:f=w93:T2)
                n80 = Select(t=Traction_Receipe_Enum."UNLOAD", s=w94, f=w93) -> (s? t:f=w92:T2)
              }
              frame "TRACTION" {
                n81 = Unbundle By Name(w121) -> ("Traction reciepe.SRR INDEX [ TRACTION]"=w144:refnum<vi>)
                n82 = Unbundle By Name(w121) -> ("Traction reciepe.BALL WEAR TRACK"=w148:refnum<vi>)
                n83 = Unbundle By Name(w121) -> ("Traction reciepe.DISC WEARTRACK"=w152:refnum<vi>)
                n84 = Unbundle By Name(w121) -> ("Traction reciepe.Traction Receipe"=w160:refnum<vi>)
                n85 = Unbundle By Name(w121) -> ("Traction reciepe.Start Index Type"=w155:refnum<vi>)
                n86 = Unbundle By Name(w121) -> ("Main Screen.Start Test Temp"=w171:refnum<vi>)
                n87 = Unbundle By Name(w121) -> ("Main Screen.STOP"=w174:refnum<vi>)
                n88 = property class="MCListbox (strict)"(reference=w160) -> (reference out=w158:refnum<vi>, error out=w159:errorcluster, "ItemNames"=w157:string[][])  [unwired: 1 in]
                n89 = property class="DigNum (strict)"(reference=w144) -> (reference out=w142:refnum<vi>, error out=w143:errorcluster, "Value"=w141:i32)  [unwired: 1 in]
                n90 = property class="DigNum (strict)"(reference=w155) -> (reference out=w154:refnum<vi>, error out=w156:errorcluster, "Value"=w153:i32)  [unwired: 1 in]
                n91 = property class="DigNum (strict)"(reference=w148) -> (reference out=w146:refnum<vi>, error out=w147:errorcluster, "Value"=w145:dbl)  [unwired: 1 in]
                n92 = property class="DigNum (strict)"(reference=w152) -> (reference out=w150:refnum<vi>, error out=w151:errorcluster, "Value"=w149:dbl)  [unwired: 1 in]
                n93 = property class="Bool (strict)"(reference=w174) -> (reference out=w176:refnum<vi>, error out=w175:errorcluster, "Value"=w173:bool)  [unwired: 1 in]
                n94 = property class="Bool (strict)"(reference=w171) -> (reference out=w169:refnum<vi>, error out=w170:errorcluster, "Value"=w172:bool)  [unwired: 1 in]
                n95 = Close Reference(reference=w176, error in (no error)=w175) -> ()  [unwired: 1 out]
                n96 = Close Reference(reference=w169, error in (no error)=w170) -> ()  [unwired: 1 out]
                n97 = Close Reference(reference=w142, error in (no error)=w143) -> ()  [unwired: 1 out]
                n98 = Close Reference(reference=w158, error in (no error)=w159) -> ()  [unwired: 1 out]
                n99 = Close Reference(reference=w154, error in (no error)=w156) -> ()  [unwired: 1 out]
                n100 = Close Reference(reference=w146, error in (no error)=w147) -> ()  [unwired: 1 out]
                n101 = Close Reference(reference=w150, error in (no error)=w151) -> ()  [unwired: 1 out]
                n102 = Index Array(array=w157, index (row)=w153) -> (element=w183:string[])  [unwired: 1 in]
                n103 = Equal?(x=w173, y=TRUE) -> (x = y?=w168:bool)
                n104 = Equal?(x=w172, y=FALSE) -> (x = y?=w167:bool)
                n105 = And(x=w168, y=w167) -> (x .and. y?=w164:bool)
                n106 = Index Array(array=w183, index=5) -> (element=w182:string)
                n107 = Index Array(array=w183, index=6) -> (element=w178:string)
                n108 = Select(t=Traction_Receipe_Enum."UNLOAD", s=w164, f=Traction_Receipe_Enum."TEMPERATURE SET" ("Enum - Menu")) -> (s? t:f=w162:T2)
                n109 = Fract/Exp String To Number(string=w178) -> (number=w181:dbl)  [unwired: 3 in, 1 out]
                n110 = Unbundle By Name(w121) -> ("Traction reciepe.Ball (mm/sec)"=w126:refnum<vi>)
                n111 = Spreadsheet String To Array(delimiter (Tab)=",", format string="", spreadsheet string=w182, array type (2D Dbl)=string[] []) -> (array=w177:string[])
                n112 = Unbundle By Name(w121) -> ("Traction reciepe.BALL SPEED (rpm)"=w133:refnum<vi>)
                n113 = Unbundle By Name(w121) -> ("Traction reciepe.Traction Size"=w140:refnum<vi>)
                n114 = Array Size(array=w177) -> (size(s)=w137:i32)
                n115 = Index Array(array=w177, index=w141) -> (element=w179:string)
                n116 = Unbundle By Name(w121) -> ("Traction reciepe.Ball (mm/sec)"=w122:refnum<vi>)
                n117 = property class="DigNum (strict)"(reference=w140, "Value"=w137) -> (reference out=w138:refnum<vi>, error out=w139:errorcluster)  [unwired: 1 in]
                n118 = Fract/Exp String To Number(string=w179) -> (number=w180:dbl)  [unwired: 3 in, 1 out]
                n119 = Close Reference(reference=w138, error in (no error)=w139) -> ()  [unwired: 1 out]
                n120 = Unbundle By Name(w121) -> ("Traction reciepe.DISC SPEED (rpm)"=w134:refnum<vi>)
                n121 = call "SSR_ENTRAINMENT VELOCITY TO MM_SEC CONVERSION.vi"("Entrainment Speed"=w181, "Initial SSR"=w180) -> ("Disc"=w120:dbl, "Ball"=w125:dbl)  [unwired: 7 in, 1 out]
                n122 = property class="DigNum (strict)"(reference=w126, "Value"=w125) -> (reference out=w128:refnum<vi>, error out=w127:errorcluster)  [unwired: 1 in]
                n123 = property class="DigNum (strict)"(reference=w122, "Value"=w120) -> (reference out=w124:refnum<vi>, error out=w123:errorcluster)  [unwired: 1 in]
                n124 = call "Rotary mm_s to rpm conversion for rotary.vi"("Wear Track Diameter"=w145, "Enter initial Velocity (m/s)  3"=w125) -> ("Initial Speed (RPM) 2"=w130:dbl)  [unwired: 7 in, 2 out]
                n125 = call "Rotary mm_s to rpm conversion for rotary.vi"("Wear Track Diameter"=w149, "Enter initial Velocity (m/s)  3"=w120) -> ("Initial Speed (RPM) 2"=w129:dbl)  [unwired: 7 in, 2 out]
                n126 = Close Reference(reference=w128, error in (no error)=w127) -> ()  [unwired: 1 out]
                n127 = Close Reference(reference=w124, error in (no error)=w123) -> ()  [unwired: 1 out]
                n128 = property class="DigNum (strict)"(reference=w133, "Value"=w130) -> (reference out=w131:refnum<vi>, error out=w132:errorcluster)  [unwired: 1 in]
                n129 = property class="DigNum (strict)"(reference=w134, "Value"=w129) -> (reference out=w136:refnum<vi>, error out=w135:errorcluster)  [unwired: 1 in]
                n130 = Close Reference(reference=w131, error in (no error)=w132) -> ()  [unwired: 1 out]
                n131 = Close Reference(reference=w136, error in (no error)=w135) -> ()  [unwired: 1 out]
              }
              frame "TEMPERATURE SET" {
                n132 = Unbundle By Name(w192) -> ("Traction reciepe.Traction Receipe"=w206:refnum<vi>)
                n133 = Unbundle By Name(w192) -> ("Traction reciepe.Start Index Type"=w201:refnum<vi>)
                n134 = Unbundle By Name(w192) -> ("Main Screen.Start Test Temp"=w217:refnum<vi>)
                n135 = Unbundle By Name(w192) -> ("Main Screen.STOP"=w220:refnum<vi>)
                n136 = property class="MCListbox (strict)"(reference=w206) -> (reference out=w204:refnum<vi>, error out=w205:errorcluster, "ItemNames"=w203:string[][])  [unwired: 1 in]
                n137 = property class="DigNum (strict)"(reference=w201) -> (reference out=w200:refnum<vi>, error out=w202:errorcluster, "Value"=w199:i32)  [unwired: 1 in]
                n138 = property class="Bool (strict)"(reference=w220) -> (reference out=w222:refnum<vi>, error out=w221:errorcluster, "Value"=w219:bool)  [unwired: 1 in]
                n139 = property class="Bool (strict)"(reference=w217) -> (reference out=w215:refnum<vi>, error out=w216:errorcluster, "Value"=w218:bool)  [unwired: 1 in]
                n140 = Close Reference(reference=w204, error in (no error)=w205) -> ()  [unwired: 1 out]
                n141 = Close Reference(reference=w200, error in (no error)=w202) -> ()  [unwired: 1 out]
                n142 = Close Reference(reference=w222, error in (no error)=w221) -> ()  [unwired: 1 out]
                n143 = Close Reference(reference=w215, error in (no error)=w216) -> ()  [unwired: 1 out]
                n144 = Index Array(array=w203, index (row)=w199) -> (element=w225:string[])  [unwired: 1 in]
                n145 = Equal?(x=w219, y=TRUE) -> (x = y?=w214:bool)
                n146 = Equal?(x=w218, y=FALSE) -> (x = y?=w213:bool)
                n147 = And(x=w214, y=w213) -> (x .and. y?=w210:bool)
                n148 = Index Array(array=w225, index=3) -> (element=w223:string)
                n149 = Select(t=Traction_Receipe_Enum."UNLOAD", s=w210, f=Traction_Receipe_Enum."CHURNING START" ("Enum - Menu")) -> (s? t:f=w208:T2)
                n150 = Fract/Exp String To Number(string=w223) -> (number=w191:dbl)  [unwired: 3 in, 1 out]
                n151 = Unbundle By Name(w192) -> ("Traction reciepe.SET TEMPERATURE"=w197:refnum<vi>)
                n152 = Unbundle By Name(w192) -> ("Main Screen.SetTmp"=w193:refnum<vi>)
                n153 = property class="DigNum (strict)"(reference=w197, "Value"=w191) -> (reference out=w196:refnum<vi>, error out=w198:errorcluster)  [unwired: 1 in]
                n154 = call "Temperature vi FGV.vi"("Enum"=Temperature_enum."write", "Set Temperature"=w191, "main ref"=w192) -> ("error out"=→"error out 3":errorcluster)  [unwired: 8 in]
                n155 = property class="DigNum (strict)"(reference=w193, "Value"=w191) -> (reference out=w190:refnum<vi>, error out=w194:errorcluster)  [unwired: 1 in]
                n156 = Close Reference(reference=w190, error in (no error)=w194) -> ()  [unwired: 1 out]
                n157 = Close Reference(reference=w196, error in (no error)=w198) -> ()  [unwired: 1 out]
              }
              frame "CHURNING START" {
                n158 = Unbundle By Name(w226) -> ("Main Screen.Start Test Temp"=w238:refnum<vi>)
                n159 = Unbundle By Name(w226) -> ("Main Screen.STOP"=w241:refnum<vi>)
                n160 = property class="Bool (strict)"(reference=w241) -> (reference out=w243:refnum<vi>, error out=w242:errorcluster, "Value"=w240:bool)  [unwired: 1 in]
                n161 = property class="Bool (strict)"(reference=w238) -> (reference out=w236:refnum<vi>, error out=w237:errorcluster, "Value"=w239:bool)  [unwired: 1 in]
                n162 = Close Reference(reference=w243, error in (no error)=w242) -> ()  [unwired: 1 out]
                n163 = Close Reference(reference=w236, error in (no error)=w237) -> ()  [unwired: 1 out]
                n164 = Equal?(x=w240, y=TRUE) -> (x = y?=w235:bool)
                n165 = Equal?(x=w239, y=FALSE) -> (x = y?=w234:bool)
                n166 = And(x=w235, y=w234) -> (x .and. y?=w231:bool)
                n167 = Select(t=Traction_Receipe_Enum."UNLOAD", s=w231, f=Traction_Receipe_Enum."TEMPERATURE REACH" ("Enum - Menu")) -> (s? t:f=w228:T2)
                n168 = call "Reciepe Disc Speed Write.vi"("Set Speed"=10.0, "main ref"=w226) -> ()  [unwired: 9 in, 1 out]
              }
              frame "TEMPERATURE REACH" {
                n169 = Unbundle By Name(w245) -> ("Traction reciepe.SET TEMPERATURE"=w250:refnum<vi>)
                n170 = Unbundle By Name(w245) -> ("Main Screen.Start Test Temp"=w263:refnum<vi>)
                n171 = Unbundle By Name(w245) -> ("Main Screen.ChamberTemp"=w246:refnum<vi>)
                n172 = Unbundle By Name(w245) -> ("Main Screen.STOP"=w266:refnum<vi>)
                n173 = property on="Property Node" class="DigNum (strict)"(reference=w246) -> (reference out=w248:refnum<vi>, error out=w247:errorcluster, "Value"=w244:dbl)  [unwired: 1 in]
                n174 = property class="DigNum (strict)"(reference=w250) -> (reference out=w252:refnum<vi>, error out=w251:errorcluster, "Value"=w249:dbl)  [unwired: 1 in]
                n175 = property class="Bool (strict)"(reference=w266) -> (reference out=w268:refnum<vi>, error out=w267:errorcluster, "Value"=w265:bool)  [unwired: 1 in]
                n176 = property class="Bool (strict)"(reference=w263) -> (reference out=w261:refnum<vi>, error out=w262:errorcluster, "Value"=w264:bool)  [unwired: 1 in]
                n177 = Close Reference(reference=w248, error in (no error)=w247) -> ()  [unwired: 1 out]
                n178 = Close Reference(reference=w268, error in (no error)=w267) -> ()  [unwired: 1 out]
                n179 = Close Reference(reference=w261, error in (no error)=w262) -> ()  [unwired: 1 out]
                n180 = Close Reference(reference=w252, error in (no error)=w251) -> ()  [unwired: 1 out]
                n181 = Greater Or Equal?(x=w244, y=w249) -> (x >= y?=w271:bool)
                n182 = Equal?(x=w265, y=TRUE) -> (x = y?=w260:bool)
                n183 = Equal?(x=w264, y=FALSE) -> (x = y?=w259:bool)
                n184 = Select(t=Traction_Receipe_Enum."CHURNING STOP" ("Enum - Menu"), s=w271, f=Traction_Receipe_Enum."TEMPERATURE REACH" ("Enum - Menu")) -> (s? t:f=w254:T2)
                n185 = And(x=w260, y=w259) -> (x .and. y?=w256:bool)
                n186 = Select(t=Traction_Receipe_Enum."UNLOAD", s=w256, f=w254) -> (s? t:f=w253:T2)
              }
              frame "CHURNING STOP" {
                n187 = Unbundle By Name(w272) -> ("Main Screen.Start Test Temp"=w284:refnum<vi>)
                n188 = Unbundle By Name(w272) -> ("Main Screen.STOP"=w287:refnum<vi>)
                n189 = property class="Bool (strict)"(reference=w287) -> (reference out=w289:refnum<vi>, error out=w288:errorcluster, "Value"=w286:bool)  [unwired: 1 in]
                n190 = property class="Bool (strict)"(reference=w284) -> (reference out=w282:refnum<vi>, error out=w283:errorcluster, "Value"=w285:bool)  [unwired: 1 in]
                n191 = Close Reference(reference=w289, error in (no error)=w288) -> ()  [unwired: 1 out]
                n192 = Close Reference(reference=w282, error in (no error)=w283) -> ()  [unwired: 1 out]
                n193 = Equal?(x=w286, y=TRUE) -> (x = y?=w281:bool)
                n194 = Equal?(x=w285, y=FALSE) -> (x = y?=w280:bool)
                n195 = And(x=w281, y=w280) -> (x .and. y?=w277:bool)
                n196 = call "Reciepe Disc Speed Write.vi"("Set Speed"=0.0, "main ref"=w272) -> ()  [unwired: 9 in, 1 out]
                n197 = Select(t=Traction_Receipe_Enum."UNLOAD", s=w277, f=Traction_Receipe_Enum."LOAD" ("Enum - Menu")) -> (s? t:f=w274:T2)
              }
              frame "LOAD" {
                n198 = Unbundle By Name(w291) -> ("Traction reciepe.Traction Receipe"=w315:refnum<vi>)
                n199 = Unbundle By Name(w291) -> ("Traction reciepe.Start Index Type"=w297:refnum<vi>)
                n200 = Unbundle By Name(w291) -> ("Main Screen.Start Test Temp"=w326:refnum<vi>)
                n201 = Unbundle By Name(w291) -> ("Main Screen.STOP"=w329:refnum<vi>)
                n202 = property class="MCListbox (strict)"(reference=w315) -> (reference out=w313:refnum<vi>, error out=w314:errorcluster, "ItemNames"=w312:string[][])  [unwired: 1 in]
                n203 = property class="DigNum (strict)"(reference=w297) -> (reference out=w296:refnum<vi>, error out=w298:errorcluster, "Value"=w295:i32)  [unwired: 1 in]
                n204 = property class="Bool (strict)"(reference=w329) -> (reference out=w331:refnum<vi>, error out=w330:errorcluster, "Value"=w328:bool)  [unwired: 1 in]
                n205 = property class="Bool (strict)"(reference=w326) -> (reference out=w324:refnum<vi>, error out=w325:errorcluster, "Value"=w327:bool)  [unwired: 1 in]
                n206 = Close Reference(reference=w331, error in (no error)=w330) -> ()  [unwired: 1 out]
                n207 = Close Reference(reference=w324, error in (no error)=w325) -> ()  [unwired: 1 out]
                n208 = Close Reference(reference=w313, error in (no error)=w314) -> ()  [unwired: 1 out]
                n209 = Close Reference(reference=w296, error in (no error)=w298) -> ()  [unwired: 1 out]
                n210 = Index Array(array=w312, index (row)=w295) -> (element=w334:string[])  [unwired: 1 in]
                n211 = Equal?(x=w328, y=TRUE) -> (x = y?=w323:bool)
                n212 = Equal?(x=w327, y=FALSE) -> (x = y?=w322:bool)
                n213 = And(x=w323, y=w322) -> (x .and. y?=w319:bool)
                n214 = Index Array(array=w334, index=4) -> (element=w333:string)
                n215 = Unbundle By Name(w291) -> ("Main Screen.Set Load (N)"=w301:refnum<vi>)
                n216 = Unbundle By Name(w291) -> ("Traction reciepe.SET LOAD"=w293:refnum<vi>)
                n217 = Select(t=Traction_Receipe_Enum."UNLOAD", s=w319, f=Traction_Receipe_Enum."LOAD REACHED" ("Enum - Menu")) -> (s? t:f=w316:T2)
                n218 = Fract/Exp String To Number(string=w333) -> (number=w290:dbl)  [unwired: 3 in, 1 out]
                n219 = property class="DigNum (strict)"(reference=w301, "Value"=w290) -> (reference out=w300:refnum<vi>, error out=w302:errorcluster)  [unwired: 1 in]
                n220 = property class="DigNum (strict)"(reference=w293, "Value"=w290) -> (reference out=w292:refnum<vi>, error out=w294:errorcluster)  [unwired: 1 in]
                n221 = Unbundle By Name(w291) -> ("Main Screen.Load En"=w311:refnum<vi>)
                n222 = Close Reference(reference=w292, error in (no error)=w294) -> ()  [unwired: 1 out]
                n223 = Close Reference(reference=w300, error in (no error)=w302) -> (error out=w299:errorcluster)
                n224 = property on="Property Node" class="Bool (strict)"(reference=w311, error in=w299, "Value"=TRUE) -> (reference out=w309:refnum<vi>, error out=w310:errorcluster)
                n225 = Unbundle By Name(w291) -> ("Main Screen.zNL 2"=w306:refnum<vi>)
                n226 = Close Reference(reference=w309, error in (no error)=w310) -> (error out=w305:errorcluster)
                n227 = property on="Property Node" class="Bool (strict)"(reference=w306, error in=w305, "DisabledEnum"=T4."Disabled and Grayed Out" ("Disabled")) -> (reference out=w308:refnum<vi>, error out=w307:errorcluster)
                n228 = Close Reference(reference=w308, error in (no error)=w307) -> ()  [unwired: 1 out]
              }
              frame "LOAD REACHED" {
                n229 = Unbundle By Name(w336) -> ("Main Screen.Start Test Temp"=w357:refnum<vi>)
                n230 = Unbundle By Name(w336) -> ("Traction reciepe.SET LOAD"=w338:refnum<vi>)
                n231 = Unbundle By Name(w336) -> ("Main Screen.NL disp 2"=w344:refnum<vi>)
                n232 = Unbundle By Name(w336) -> ("Main Screen.STOP"=w360:refnum<vi>)
                n233 = property class="DigNum (strict)"(reference=w344) -> (reference out=w346:refnum<vi>, error out=w345:errorcluster, "Value"=w343:dbl)  [unwired: 1 in]
                n234 = property class="DigNum (strict)"(reference=w338) -> (reference out=w340:refnum<vi>, error out=w339:errorcluster, "Value"=w337:dbl)  [unwired: 1 in]
                n235 = property class="Bool (strict)"(reference=w360) -> (reference out=w362:refnum<vi>, error out=w361:errorcluster, "Value"=w359:bool)  [unwired: 1 in]
                n236 = property class="Bool (strict)"(reference=w357) -> (reference out=w355:refnum<vi>, error out=w356:errorcluster, "Value"=w358:bool)  [unwired: 1 in]
                n237 = Close Reference(reference=w362, error in (no error)=w361) -> ()  [unwired: 1 out]
                n238 = Close Reference(reference=w355, error in (no error)=w356) -> ()  [unwired: 1 out]
                n239 = Close Reference(reference=w346, error in (no error)=w345) -> ()  [unwired: 1 out]
                n240 = Close Reference(reference=w340, error in (no error)=w339) -> ()  [unwired: 1 out]
                n241 = Equal?(x=w359, y=TRUE) -> (x = y?=w354:bool)
                n242 = Equal?(x=w358, y=FALSE) -> (x = y?=w353:bool)
                n243 = Subtract(x=w337, y=0.4) -> (x-y=w342:dbl)
                n244 = Greater Or Equal?(x=w343, y=w342) -> (x >= y?=w335:bool)
                n245 = And(x=w354, y=w353) -> (x .and. y?=w350:bool)
                n246 = Select(t=Traction_Receipe_Enum."SRR SET" ("Enum - Menu"), s=w335, f=Traction_Receipe_Enum."LOAD REACHED" ("Enum - Menu")) -> (s? t:f=w348:T2)
                n247 = case shown="True" w335 {
                  tunnel: w336 -> [_ w365]
                  frame False {
                  }
                  frame True {
                    n248 = Unbundle By Name(w365) -> ("Traction reciepe.Traction Receipe Update Details"=w377:refnum<vi>)
                    n249 = Unbundle By Name(w365) -> ("Main Screen.Depthz"=w369:refnum<vi>)
                    n250 = Unbundle By Name(w365) -> ("Main Screen.zFF"=w373:refnum<vi>)
                    n251 = property class="Bool (strict)"(reference=w377, "Value"=TRUE) -> (reference out=w376:refnum<vi>, error out=w378:errorcluster)  [unwired: 1 in]
                    n252 = property class="Bool (strict)"(reference=w373, "DisabledEnum"=T4."Disabled and Grayed Out" ("Disabled"), "Value"=TRUE) -> (reference out=w374:refnum<vi>, error out=w372:errorcluster)  [unwired: 1 in]
                    n253 = property class="Bool (strict)"(reference=w369, "Value"=TRUE) -> (reference out=w367:refnum<vi>, error out=w368:errorcluster)  [unwired: 1 in]
                    n254 = Close Reference(reference=w376, error in (no error)=w378) -> ()  [unwired: 1 out]
                    n255 = Close Reference(reference=w374, error in (no error)=w372) -> ()  [unwired: 1 out]
                    n256 = Close Reference(reference=w367, error in (no error)=w368) -> ()  [unwired: 1 out]
                  }
                }
                n257 = Select(t=Traction_Receipe_Enum."UNLOAD", s=w350, f=w348) -> (s? t:f=w347:T2)
              }
              frame "SRR SET" {
                w478 = TRUE ("PAUSE")
                n258 = call "ELAPSED TIMER VI FOR SRR TRACTION.vi"("RESET"=w478, "PAUSE"=w478) -> ()  [unwired: 7 in, 3 out]
                n259 = Unbundle By Name(w383) -> ("Traction reciepe.SRR INDEX [ TRACTION]"=w421:refnum<vi>)
                n260 = Unbundle By Name(w383) -> ("Traction reciepe.BALL WEAR TRACK"=w437:refnum<vi>)
                n261 = Unbundle By Name(w383) -> ("Traction reciepe.DISC WEARTRACK"=w441:refnum<vi>)
                n262 = Unbundle By Name(w383) -> ("Traction reciepe.Traction Receipe"=w451:refnum<vi>)
                n263 = Unbundle By Name(w383) -> ("Traction reciepe.Start Index Type"=w444:refnum<vi>)
                n264 = Unbundle By Name(w383) -> ("Main Screen.Start Test Temp"=w462:refnum<vi>)
                n265 = Unbundle By Name(w383) -> ("Main Screen.STOP"=w465:refnum<vi>)
                n266 = property class="MCListbox (strict)"(reference=w451) -> (reference out=w449:refnum<vi>, error out=w450:errorcluster, "ItemNames"=w448:string[][])  [unwired: 1 in]
                n267 = property class="DigNum (strict)"(reference=w437) -> (reference out=w435:refnum<vi>, error out=w436:errorcluster, "Value"=w434:dbl)  [unwired: 1 in]
                n268 = property class="DigNum (strict)"(reference=w421) -> (reference out=w419:refnum<vi>, error out=w420:errorcluster, "Value"=w418:i32)  [unwired: 1 in]
                n269 = property class="DigNum (strict)"(reference=w444) -> (reference out=w443:refnum<vi>, error out=w445:errorcluster, "Value"=w442:i32)  [unwired: 1 in]
                n270 = property class="DigNum (strict)"(reference=w441) -> (reference out=w439:refnum<vi>, error out=w440:errorcluster, "Value"=w438:dbl)  [unwired: 1 in]
                n271 = property class="Bool (strict)"(reference=w465) -> (reference out=w467:refnum<vi>, error out=w466:errorcluster, "Value"=w464:bool)  [unwired: 1 in]
                n272 = property class="Bool (strict)"(reference=w462) -> (reference out=w460:refnum<vi>, error out=w461:errorcluster, "Value"=w463:bool)  [unwired: 1 in]
                n273 = Close Reference(reference=w467, error in (no error)=w466) -> ()  [unwired: 1 out]
                n274 = Close Reference(reference=w460, error in (no error)=w461) -> ()  [unwired: 1 out]
                n275 = Close Reference(reference=w435, error in (no error)=w436) -> ()  [unwired: 1 out]
                n276 = Close Reference(reference=w419, error in (no error)=w420) -> ()  [unwired: 1 out]
                n277 = Close Reference(reference=w449, error in (no error)=w450) -> ()  [unwired: 1 out]
                n278 = Close Reference(reference=w443, error in (no error)=w445) -> ()  [unwired: 1 out]
                n279 = Close Reference(reference=w439, error in (no error)=w440) -> ()  [unwired: 1 out]
                n280 = Index Array(array=w448, index (row)=w442) -> (element=w477:string[])  [unwired: 1 in]
                n281 = Equal?(x=w464, y=TRUE) -> (x = y?=w459:bool)
                n282 = Equal?(x=w463, y=FALSE) -> (x = y?=w458:bool)
                n283 = And(x=w459, y=w458) -> (x .and. y?=w455:bool)
                n284 = Index Array(array=w477, index=5) -> (element=w476:string)
                n285 = Index Array(array=w477, index=6) -> (element=w474:string)
                n286 = Unbundle By Name(w383) -> ("Traction reciepe.SET entrainment Velocity"=w429:refnum<vi>)
                n287 = Select(t=Traction_Receipe_Enum."UNLOAD", s=w455, f=Traction_Receipe_Enum."SRR WAIT" ("Enum - Menu")) -> (s? t:f=w452:T2)
                n288 = Fract/Exp String To Number(string=w474) -> (number=w426:dbl)  [unwired: 3 in, 1 out]
                n289 = property class="DigNum (strict)"(reference=w429, "Value"=w426) -> (reference out=w427:refnum<vi>, error out=w428:errorcluster)  [unwired: 1 in]
                n290 = Spreadsheet String To Array(delimiter (Tab)=",", format string="", spreadsheet string=w476, array type (2D Dbl)=string[] []) -> (array=w473:string[])
                n291 = Close Reference(reference=w427, error in (no error)=w428) -> ()  [unwired: 1 out]
                n292 = Unbundle By Name(w383) -> ("Traction reciepe.BALL SET RPM"=w407:refnum<vi>)
                n293 = Unbundle By Name(w383) -> ("Traction reciepe.Traction Size"=w425:refnum<vi>)
                n294 = Array Size(array=w473) -> (size(s)=w422:i32)
                n295 = Index Array(array=w473, index=w418) -> (element=w475:string)
                n296 = Unbundle By Name(w383) -> ("Traction reciepe.DISC SET RPM"=w410:refnum<vi>)
                n297 = property class="DigNum (strict)"(reference=w425, "Value"=w422) -> (reference out=w423:refnum<vi>, error out=w424:errorcluster)  [unwired: 1 in]
                n298 = Unbundle By Name(w383) -> ("Traction reciepe.SET SRR"=w433:refnum<vi>)
                n299 = Fract/Exp String To Number(string=w475) -> (number=w430:dbl)  [unwired: 3 in, 1 out]
                n300 = Unbundle By Name(w383) -> ("Traction Control.Disc Motion Direction:"=w397:refnum<vi>)
                n301 = property class="DigNum (strict)"(reference=w433, "Value"=w430) -> (reference out=w431:refnum<vi>, error out=w432:errorcluster)  [unwired: 1 in]
                n302 = Close Reference(reference=w423, error in (no error)=w424) -> ()  [unwired: 1 out]
                n303 = Unbundle By Name(w383) -> ("Traction reciepe.Ball (mm/sec)"=w402:refnum<vi>)
                n304 = Divide(x=w430, y=100.0) -> (x/y=w447:dbl)
                n305 = property class="Ring (strict)"(reference=w397) -> (reference out=w395:refnum<vi>, error out=w396:errorcluster, "Value"=w394:u16)  [unwired: 1 in]
                n306 = Close Reference(reference=w431, error in (no error)=w432) -> ()  [unwired: 1 out]
                n307 = Unbundle By Name(w383) -> ("Traction reciepe.BALL SPEED (rpm)"=w400:refnum<vi>)
                n308 = Unbundle By Name(w383) -> ("Traction reciepe.DISC SPEED (rpm)"=w411:refnum<vi>)
                n309 = Unbundle By Name(w383) -> ("Traction reciepe.Disc (mm/sec)"=w417:refnum<vi>)
                n310 = call "SSR_ENTRAINMENT VELOCITY TO MM_SEC CONVERSION.vi"("Entrainment Speed"=w426, "Initial SSR"=w447) -> ("Disc"=w414:dbl, "Ball"=w401:dbl)  [unwired: 7 in, 1 out]
                n311 = Close Reference(reference=w395, error in (no error)=w396) -> ()  [unwired: 1 out]
                n312 = Equal?(x=w394, y=u16 0) -> (x = y?=w392:bool)
                n313 = property class="DigNum (strict)"(reference=w402, "Value"=w401) -> (reference out=w404:refnum<vi>, error out=w403:errorcluster)  [unwired: 1 in]
                n314 = property class="DigNum (strict)"(reference=w417, "Value"=w414) -> (reference out=w415:refnum<vi>, error out=w416:errorcluster)  [unwired: 1 in]
                n315 = call "Rotary mm_s to rpm conversion for rotary.vi"("Wear Track Diameter"=w434, "Enter initial Velocity (m/s)  3"=w401) -> ("Initial Speed (RPM) 2"=w381:dbl)  [unwired: 7 in, 2 out]
                n316 = call "Rotary mm_s to rpm conversion for rotary.vi"("Wear Track Diameter"=w438, "Enter initial Velocity (m/s)  3"=w414) -> ("Initial Speed (RPM) 2"=w391:dbl)  [unwired: 7 in, 2 out]
                n317 = Negate(x=w391) -> (-x=w390:dbl)
                n318 = Select(t=w391, s=w392, f=w390) -> (s? t:f=w389:dbl)
                n319 = call "Reciepe Disc Speed Write.vi"("Set Speed"=w389, "main ref"=w383) -> ()  [unwired: 9 in, 1 out]
                n320 = Close Reference(reference=w404, error in (no error)=w403) -> ()  [unwired: 1 out]
                n321 = Close Reference(reference=w415, error in (no error)=w416) -> ()  [unwired: 1 out]
                n322 = property class="DigNum (strict)"(reference=w407, "Value"=w381) -> (reference out=w405:refnum<vi>, error out=w406:errorcluster)  [unwired: 1 in]
                n323 = property class="DigNum (strict)"(reference=w400, "Value"=w381) -> (reference out=w398:refnum<vi>, error out=w399:errorcluster)  [unwired: 1 in]
                n324 = property class="DigNum (strict)"(reference=w411, "Value"=w391) -> (reference out=w413:refnum<vi>, error out=w412:errorcluster)  [unwired: 1 in]
                n325 = property class="DigNum (strict)"(reference=w410, "Value"=w391) -> (reference out=w408:refnum<vi>, error out=w409:errorcluster)  [unwired: 1 in]
                n326 = Close Reference(reference=w405, error in (no error)=w406) -> ()  [unwired: 1 out]
                n327 = Close Reference(reference=w398, error in (no error)=w399) -> ()  [unwired: 1 out]
                n328 = Close Reference(reference=w413, error in (no error)=w412) -> ()  [unwired: 1 out]
                n329 = Close Reference(reference=w408, error in (no error)=w409) -> ()  [unwired: 1 out]
                n330 = Unbundle By Name(w383) -> ("Traction Control.Ball Motion Direction :"=w388:refnum<vi>)
                n331 = property class="Ring (strict)"(reference=w388) -> (reference out=w386:refnum<vi>, error out=w387:errorcluster, "Value"=w385:u16)  [unwired: 1 in]
                n332 = Close Reference(reference=w386, error in (no error)=w387) -> ()  [unwired: 1 out]
                n333 = Equal?(x=w385, y=u16 0) -> (x = y?=w380:bool)
                n334 = Negate(x=w381) -> (-x=w382:dbl)
                n335 = Select(t=w381, s=w380, f=w382) -> (s? t:f=w379:dbl)
                n336 = call "Reciepe Ball Speed Write.vi"("Set Speed"=w379, "main ref"=w383) -> ()  [unwired: 9 in, 1 out]
              }
              frame "SRR WAIT" {
                w512 = FALSE ("PAUSE")
                n337 = Unbundle By Name(w480) -> ("Traction reciepe.Traction Receipe"=w491:refnum<vi>)
                n338 = Unbundle By Name(w480) -> ("Traction reciepe.Start Index Type"=w486:refnum<vi>)
                n339 = Unbundle By Name(w480) -> ("Traction reciepe.ELAPSED TIMER"=w483:refnum<vi>)
                n340 = Unbundle By Name(w480) -> ("Main Screen.Start Test Temp"=w502:refnum<vi>)
                n341 = Unbundle By Name(w480) -> ("Main Screen.STOP"=w505:refnum<vi>)
                n342 = property class="MCListbox (strict)"(reference=w491) -> (reference out=w489:refnum<vi>, error out=w490:errorcluster, "ItemNames"=w488:string[][])  [unwired: 1 in]
                n343 = property class="DigNum (strict)"(reference=w486) -> (reference out=w485:refnum<vi>, error out=w487:errorcluster, "Value"=w484:i32)  [unwired: 1 in]
                n344 = property class="Bool (strict)"(reference=w505) -> (reference out=w507:refnum<vi>, error out=w506:errorcluster, "Value"=w504:bool)  [unwired: 1 in]
                n345 = property class="Bool (strict)"(reference=w502) -> (reference out=w500:refnum<vi>, error out=w501:errorcluster, "Value"=w503:bool)  [unwired: 1 in]
                n346 = Close Reference(reference=w507, error in (no error)=w506) -> ()  [unwired: 1 out]
                n347 = Close Reference(reference=w500, error in (no error)=w501) -> ()  [unwired: 1 out]
                n348 = Close Reference(reference=w489, error in (no error)=w490) -> ()  [unwired: 1 out]
                n349 = Close Reference(reference=w485, error in (no error)=w487) -> ()  [unwired: 1 out]
                n350 = Index Array(array=w488, index (row)=w484) -> (element=w515:string[])  [unwired: 1 in]
                n351 = Equal?(x=w504, y=TRUE) -> (x = y?=w499:bool)
                n352 = Equal?(x=w503, y=FALSE) -> (x = y?=w498:bool)
                n353 = And(x=w499, y=w498) -> (x .and. y?=w495:bool)
                n354 = Index Array(array=w515, index=7) -> (element=w514:string)
                n355 = Fract/Exp String To Number(string=w514) -> (number=w511:dbl)  [unwired: 3 in, 1 out]
                n356 = call "ELAPSED TIMER VI FOR SRR TRACTION.vi"("TARGET"=w511, "RESET"=w512, "PAUSE"=w512) -> ("ELAPSED INDICATION"=w510:bool, "ELAPSED TIMER"=w479:dbl)  [unwired: 6 in, 1 out]
                n357 = property class="DigNum (strict)"(reference=w483, "Value"=w479) -> (reference out=w481:refnum<vi>, error out=w482:errorcluster)  [unwired: 1 in]
                n358 = Select(t=Traction_Receipe_Enum."SRR INCREMENT" ("Enum - Menu"), s=w510, f=Traction_Receipe_Enum."SRR WAIT") -> (s? t:f=w493:T2)
                n359 = Close Reference(reference=w481, error in (no error)=w482) -> ()  [unwired: 1 out]
                n360 = Select(t=Traction_Receipe_Enum."UNLOAD", s=w495, f=w493) -> (s? t:f=w492:T2)
              }
              frame "SRR INCREMENT" {
                n361 = Unbundle By Name(w516) -> ("Main Screen.Start Test Temp"=w527:refnum<vi>)
                n362 = Unbundle By Name(w516) -> ("Main Screen.STOP"=w530:refnum<vi>)
                n363 = flat-sequence {
                  tunnel: w516 -> [w539]
                  tunnel: [w552] -> w518
                  tunnel: w516 -> [w550]
                  tunnel: w516 -> [w542]
                  frame #0 {
                    n364 = Unbundle By Name(w539) -> ("Traction reciepe.SRR INDEX [ TRACTION]"=w540:refnum<vi>)
                    n365 = property class="DigNum (strict)"(reference=w540) -> (reference out=w536:refnum<vi>, error out=w535:errorcluster, "Value"=w534:i32)  [unwired: 1 in]
                    n366 = Increment(x=w534) -> (x+1=w533:i32)
                    n367 = property class="DigNum (strict)"(reference=w536, error in=w535, "Value"=w533) -> (reference out=w537:refnum<vi>, error out=w538:errorcluster)
                    n368 = Close Reference(reference=w537, error in (no error)=w538) -> ()  [unwired: 1 out]
                  }
                  frame #1 {
                    n369 = Unbundle By Name(w542) -> ("Traction reciepe.SRR INDEX [ TRACTION]"=w547:refnum<vi>)
                    n370 = Unbundle By Name(w542) -> ("Traction reciepe.Traction Size"=w545:refnum<vi>)
                    n371 = property class="DigNum (strict)"(reference=w547) -> (reference out=w549:refnum<vi>, error out=w548:errorcluster, "Value"=w546:i32)  [unwired: 1 in]
                    n372 = property class="DigNum (strict)"(reference=w545) -> (reference out=w543:refnum<vi>, error out=w544:errorcluster, "Value"=w541:i32)  [unwired: 1 in]
                    n373 = Close Reference(reference=w549, error in (no error)=w548) -> ()  [unwired: 1 out]
                    n374 = Close Reference(reference=w543, error in (no error)=w544) -> ()  [unwired: 1 out]
                    n375 = Greater Or Equal?(x=w546, y=w541) -> (x >= y?=w551:bool)
                    n376 = case shown="True" w551 {
                      tunnel: w550 -> [_ w556]
                      frame False {
                      }
                      frame True {
                        n377 = Unbundle By Name(w556) -> ("Traction reciepe.SRR INDEX [ TRACTION]"=w558:refnum<vi>)
                        n378 = Unbundle By Name(w556) -> ("Traction reciepe.Start Index Type"=w566:refnum<vi>)
                        n379 = Unbundle By Name(w556) -> ("Traction reciepe.Start Index Type"=w562:refnum<vi>)
                        n380 = property class="DigNum (strict)"(reference=w562) -> (reference out=w561:refnum<vi>, error out=w563:errorcluster, "Value"=w560:i32)  [unwired: 1 in]
                        n381 = property class="DigNum (strict)"(reference=w558, "Value"=0 ("SRR INDEX [ TRACTION]")) -> (reference out=w557:refnum<vi>, error out=w559:errorcluster)  [unwired: 1 in]
                        n382 = Close Reference(reference=w561, error in (no error)=w563) -> ()  [unwired: 1 out]
                        n383 = Close Reference(reference=w557, error in (no error)=w559) -> ()  [unwired: 1 out]
                        n384 = Increment(x=w560) -> (x+1=w564:i32)
                        n385 = property class="DigNum (strict)"(reference=w566, "Value"=w564) -> (reference out=w565:refnum<vi>, error out=w567:errorcluster)  [unwired: 1 in]
                        n386 = Close Reference(reference=w565, error in (no error)=w567) -> ()  [unwired: 1 out]
                      }
                    }
                    n387 = Select(t=Traction_Receipe_Enum."START" ("Enum - Menu"), s=w551, f=Traction_Receipe_Enum."SRR SET" ("Enum - Menu")) -> (s? t:f=w552:T2)
                  }
                }
                n388 = property class="Bool (strict)"(reference=w530) -> (reference out=w532:refnum<vi>, error out=w531:errorcluster, "Value"=w529:bool)  [unwired: 1 in]
                n389 = property class="Bool (strict)"(reference=w527) -> (reference out=w525:refnum<vi>, error out=w526:errorcluster, "Value"=w528:bool)  [unwired: 1 in]
                n390 = Close Reference(reference=w532, error in (no error)=w531) -> ()  [unwired: 1 out]
                n391 = Close Reference(reference=w525, error in (no error)=w526) -> ()  [unwired: 1 out]
                n392 = Equal?(x=w529, y=TRUE) -> (x = y?=w524:bool)
                n393 = Equal?(x=w528, y=FALSE) -> (x = y?=w523:bool)
                n394 = And(x=w524, y=w523) -> (x .and. y?=w520:bool)
                n395 = Select(t=Traction_Receipe_Enum."UNLOAD", s=w520, f=w518) -> (s? t:f=w517:T2)
              }
              frame "STRIBECK" {
                n396 = Unbundle By Name(w570) -> ("Traction reciepe.SRR INDEX [ STRIBECK]"=w602:refnum<vi>)
                n397 = Unbundle By Name(w570) -> ("Traction reciepe.BALL WEAR TRACK"=w612:refnum<vi>)
                n398 = Unbundle By Name(w570) -> ("Traction reciepe.DISC WEARTRACK"=w616:refnum<vi>)
                n399 = Unbundle By Name(w570) -> ("Traction reciepe.Traction Receipe"=w626:refnum<vi>)
                n400 = Unbundle By Name(w570) -> ("Traction reciepe.Start Index Type"=w619:refnum<vi>)
                n401 = Unbundle By Name(w570) -> ("Main Screen.Start Test Temp"=w637:refnum<vi>)
                n402 = Unbundle By Name(w570) -> ("Main Screen.STOP"=w640:refnum<vi>)
                n403 = property class="MCListbox (strict)"(reference=w626) -> (reference out=w624:refnum<vi>, error out=w625:errorcluster, "ItemNames"=w623:string[][])  [unwired: 1 in]
                n404 = property class="DigNum (strict)"(reference=w612) -> (reference out=w610:refnum<vi>, error out=w611:errorcluster, "Value"=w609:dbl)  [unwired: 1 in]
                n405 = property class="DigNum (strict)"(reference=w602) -> (reference out=w604:refnum<vi>, error out=w603:errorcluster, "Value"=w601:i32)  [unwired: 1 in]
                n406 = property class="DigNum (strict)"(reference=w619) -> (reference out=w618:refnum<vi>, error out=w620:errorcluster, "Value"=w617:i32)  [unwired: 1 in]
                n407 = property class="DigNum (strict)"(reference=w616) -> (reference out=w614:refnum<vi>, error out=w615:errorcluster, "Value"=w613:dbl)  [unwired: 1 in]
                n408 = property class="Bool (strict)"(reference=w640) -> (reference out=w642:refnum<vi>, error out=w641:errorcluster, "Value"=w639:bool)  [unwired: 1 in]
                n409 = property class="Bool (strict)"(reference=w637) -> (reference out=w635:refnum<vi>, error out=w636:errorcluster, "Value"=w638:bool)  [unwired: 1 in]
                n410 = Close Reference(reference=w642, error in (no error)=w641) -> ()  [unwired: 1 out]
                n411 = Close Reference(reference=w635, error in (no error)=w636) -> ()  [unwired: 1 out]
                n412 = Close Reference(reference=w610, error in (no error)=w611) -> ()  [unwired: 1 out]
                n413 = Close Reference(reference=w604, error in (no error)=w603) -> ()  [unwired: 1 out]
                n414 = Close Reference(reference=w624, error in (no error)=w625) -> ()  [unwired: 1 out]
                n415 = Close Reference(reference=w618, error in (no error)=w620) -> ()  [unwired: 1 out]
                n416 = Close Reference(reference=w614, error in (no error)=w615) -> ()  [unwired: 1 out]
                n417 = Index Array(array=w623, index (row)=w617) -> (element=w649:string[])  [unwired: 1 in]
                n418 = Equal?(x=w639, y=TRUE) -> (x = y?=w634:bool)
                n419 = Equal?(x=w638, y=FALSE) -> (x = y?=w633:bool)
                n420 = And(x=w634, y=w633) -> (x .and. y?=w630:bool)
                n421 = Index Array(array=w649, index=6) -> (element=w648:string)
                n422 = Index Array(array=w649, index=5) -> (element=w652:string)
                n423 = Unbundle By Name(w570) -> ("Traction reciepe.SET SRR"=w598:refnum<vi>)
                n424 = Select(t=Traction_Receipe_Enum."UNLOAD", s=w630, f=Traction_Receipe_Enum."SPEED SET" ("Enum - Menu")) -> (s? t:f=w627:T2)
                n425 = Fract/Exp String To Number(string=w652) -> (number=w597:dbl)  [unwired: 3 in, 1 out]
                n426 = property class="DigNum (strict)"(reference=w598, "Value"=w597) -> (reference out=w600:refnum<vi>, error out=w599:errorcluster)  [unwired: 1 in]
                n427 = Spreadsheet String To Array(delimiter (Tab)=",", format string="", spreadsheet string=w648, array type (2D Dbl)=string[] []) -> (array=w650:string[])
                n428 = Close Reference(reference=w600, error in (no error)=w599) -> ()  [unwired: 1 out]
                n429 = Unbundle By Name(w570) -> ("Traction reciepe.Stribeck Size"=w594:refnum<vi>)
                n430 = Array Size(array=w650) -> (size(s)=w593:i32)
                n431 = Index Array(array=w650, index=w601) -> (element=w651:string)
                n432 = Divide(x=w597, y=100.0) -> (x/y=w622:dbl)
                n433 = Unbundle By Name(w570) -> ("Traction reciepe.SET entrainment Velocity"=w608:refnum<vi>)
                n434 = Unbundle By Name(w570) -> ("Traction reciepe.DISC SPEED (rpm)"=w590:refnum<vi>)
                n435 = property class="DigNum (strict)"(reference=w594, "Value"=w593) -> (reference out=w596:refnum<vi>, error out=w595:errorcluster)  [unwired: 1 in]
                n436 = Unbundle By Name(w570) -> ("Traction Control.Disc Motion Direction:"=w586:refnum<vi>)
                n437 = Fract/Exp String To Number(string=w651) -> (number=w605:dbl)  [unwired: 3 in, 1 out]
                n438 = property class="DigNum (strict)"(reference=w608, "Value"=w605) -> (reference out=w606:refnum<vi>, error out=w607:errorcluster)  [unwired: 1 in]
                n439 = Close Reference(reference=w596, error in (no error)=w595) -> ()  [unwired: 1 out]
                n440 = property class="Ring (strict)"(reference=w586) -> (reference out=w584:refnum<vi>, error out=w585:errorcluster, "Value"=w583:u16)  [unwired: 1 in]
                n441 = call "ENTRAINMENT VELOCITY_SSR TO MM_SEC CONVERSION.vi"("SSR"=w622, "INITIAL Entrainment Speed"=w605) -> ("Disc"=w654:dbl, "Ball"=w653:dbl)  [unwired: 7 in, 1 out]
                n442 = Close Reference(reference=w606, error in (no error)=w607) -> ()  [unwired: 1 out]
                n443 = Unbundle By Name(w570) -> ("Traction reciepe.BALL SPEED (rpm)"=w589:refnum<vi>)
                n444 = Close Reference(reference=w584, error in (no error)=w585) -> ()  [unwired: 1 out]
                n445 = Equal?(x=w583, y=u16 0) -> (x = y?=w581:bool)
                n446 = call "Rotary mm_s to rpm conversion for rotary.vi"("Wear Track Diameter"=w609, "Enter initial Velocity (m/s)  3"=w653) -> ("Initial Speed (RPM) 2"=w569:dbl)  [unwired: 7 in, 2 out]
                n447 = call "Rotary mm_s to rpm conversion for rotary.vi"("Wear Track Diameter"=w613, "Enter initial Velocity (m/s)  3"=w654) -> ("Initial Speed (RPM) 2"=w579:dbl)  [unwired: 7 in, 2 out]
                n448 = Negate(x=w579) -> (-x=w580:dbl)
                n449 = Select(t=w579, s=w581, f=w580) -> (s? t:f=w578:dbl)
                n450 = property class="DigNum (strict)"(reference=w589, "Value"=w569) -> (reference out=w587:refnum<vi>, error out=w588:errorcluster)  [unwired: 1 in]
                n451 = property class="DigNum (strict)"(reference=w590, "Value"=w579) -> (reference out=w592:refnum<vi>, error out=w591:errorcluster)  [unwired: 1 in]
                n452 = call "Reciepe Disc Speed Write.vi"("Set Speed"=w578, "main ref"=w570) -> ()  [unwired: 9 in, 1 out]
                n453 = Unbundle By Name(w570) -> ("Traction Control.Ball Motion Direction :"=w577:refnum<vi>)
                n454 = Close Reference(reference=w587, error in (no error)=w588) -> ()  [unwired: 1 out]
                n455 = Close Reference(reference=w592, error in (no error)=w591) -> ()  [unwired: 1 out]
                n456 = property class="Ring (strict)"(reference=w577) -> (reference out=w575:refnum<vi>, error out=w576:errorcluster, "Value"=w574:u16)  [unwired: 1 in]
                n457 = Close Reference(reference=w575, error in (no error)=w576) -> ()  [unwired: 1 out]
                n458 = Equal?(x=w574, y=u16 0) -> (x = y?=w571:bool)
                n459 = Negate(x=w569) -> (-x=w572:dbl)
                n460 = Select(t=w569, s=w571, f=w572) -> (s? t:f=w568:dbl)
                n461 = call "Reciepe Ball Speed Write.vi"("Set Speed"=w568, "main ref"=w570) -> ()  [unwired: 9 in, 1 out]
              }
              frame "SPEED SET" {
                w672 = TRUE ("PAUSE")
                n462 = Unbundle By Name(w657) -> ("Main Screen.Start Test Temp"=w666:refnum<vi>)
                n463 = Unbundle By Name(w657) -> ("Main Screen.STOP"=w669:refnum<vi>)
                n464 = property class="Bool (strict)"(reference=w669) -> (reference out=w671:refnum<vi>, error out=w670:errorcluster, "Value"=w668:bool)  [unwired: 1 in]
                n465 = property class="Bool (strict)"(reference=w666) -> (reference out=w664:refnum<vi>, error out=w665:errorcluster, "Value"=w667:bool)  [unwired: 1 in]
                n466 = Close Reference(reference=w671, error in (no error)=w670) -> ()  [unwired: 1 out]
                n467 = Close Reference(reference=w664, error in (no error)=w665) -> ()  [unwired: 1 out]
                n468 = Equal?(x=w668, y=TRUE) -> (x = y?=w663:bool)
                n469 = Equal?(x=w667, y=FALSE) -> (x = y?=w662:bool)
                n470 = And(x=w663, y=w662) -> (x .and. y?=w659:bool)
                n471 = Select(t=Traction_Receipe_Enum."UNLOAD", s=w659, f=Traction_Receipe_Enum."SPEED WAIT" ("Enum - Menu")) -> (s? t:f=w655:T2)
                n472 = call "ELAPSED TIMER VI FOR MM_SEC TRACTION.vi"("RESET"=w672, "PAUSE"=w672) -> ()  [unwired: 7 in, 3 out]
              }
              frame "SPEED WAIT" {
                w705 = FALSE ("PAUSE")
                n473 = Unbundle By Name(w674) -> ("Traction reciepe.Traction Receipe"=w685:refnum<vi>)
                n474 = Unbundle By Name(w674) -> ("Traction reciepe.Start Index Type"=w680:refnum<vi>)
                n475 = Unbundle By Name(w674) -> ("Traction reciepe.ELAPSED TIMER"=w677:refnum<vi>)
                n476 = Unbundle By Name(w674) -> ("Main Screen.Start Test Temp"=w696:refnum<vi>)
                n477 = Unbundle By Name(w674) -> ("Main Screen.STOP"=w699:refnum<vi>)
                n478 = property class="MCListbox (strict)"(reference=w685) -> (reference out=w683:refnum<vi>, error out=w684:errorcluster, "ItemNames"=w682:string[][])  [unwired: 1 in]
                n479 = property class="DigNum (strict)"(reference=w680) -> (reference out=w679:refnum<vi>, error out=w681:errorcluster, "Value"=w678:i32)  [unwired: 1 in]
                n480 = property class="Bool (strict)"(reference=w699) -> (reference out=w701:refnum<vi>, error out=w700:errorcluster, "Value"=w698:bool)  [unwired: 1 in]
                n481 = property class="Bool (strict)"(reference=w696) -> (reference out=w694:refnum<vi>, error out=w695:errorcluster, "Value"=w697:bool)  [unwired: 1 in]
                n482 = Close Reference(reference=w701, error in (no error)=w700) -> ()  [unwired: 1 out]
                n483 = Close Reference(reference=w694, error in (no error)=w695) -> ()  [unwired: 1 out]
                n484 = Close Reference(reference=w683, error in (no error)=w684) -> ()  [unwired: 1 out]
                n485 = Close Reference(reference=w679, error in (no error)=w681) -> ()  [unwired: 1 out]
                n486 = Index Array(array=w682, index (row)=w678) -> (element=w709:string[])  [unwired: 1 in]
                n487 = Equal?(x=w698, y=TRUE) -> (x = y?=w693:bool)
                n488 = Equal?(x=w697, y=FALSE) -> (x = y?=w692:bool)
                n489 = And(x=w693, y=w692) -> (x .and. y?=w689:bool)
                n490 = Index Array(array=w709, index=7) -> (element=w708:string)
                n491 = Fract/Exp String To Number(string=w708) -> (number=w706:dbl)  [unwired: 3 in, 1 out]
                n492 = call "ELAPSED TIMER VI FOR MM_SEC TRACTION.vi"("TARGET"=w706, "RESET"=w705, "PAUSE"=w705) -> ("ELAPSED INDICATION"=w702:bool, "ELAPSED TIMER"=w673:dbl)  [unwired: 6 in, 1 out]
                n493 = property class="DigNum (strict)"(reference=w677, "Value"=w673) -> (reference out=w675:refnum<vi>, error out=w676:errorcluster)  [unwired: 1 in]
                n494 = Select(t=Traction_Receipe_Enum."SPEED INCREMENT" ("Enum - Menu"), s=w702, f=Traction_Receipe_Enum."SPEED WAIT") -> (s? t:f=w687:T2)
                n495 = Close Reference(reference=w675, error in (no error)=w676) -> ()  [unwired: 1 out]
                n496 = Select(t=Traction_Receipe_Enum."UNLOAD", s=w689, f=w687) -> (s? t:f=w686:T2)
              }
              frame "SPEED INCREMENT" {
                n497 = Unbundle By Name(w710) -> ("Traction reciepe.Traction Receipe"=w715:refnum<vi>)
                n498 = Unbundle By Name(w710) -> ("Main Screen.Start Test Temp"=w726:refnum<vi>)
                n499 = Unbundle By Name(w710) -> ("Main Screen.STOP"=w729:refnum<vi>)
                n500 = flat-sequence {
                  tunnel: w710 -> [w733]
                  tunnel: [w752] -> w732
                  tunnel: w710 -> [w742]
                  tunnel: [w742] -> w711
                  tunnel: [w780] -> w717
                  tunnel: w732 -> [w779]
                  tunnel: w712 -> [w777]
                  tunnel: w711 -> [w773]
                  frame #0 {
                    n501 = Unbundle By Name(w733) -> ("Traction reciepe.SRR INDEX [ STRIBECK]"=w734:refnum<vi>)
                    n502 = property class="DigNum (strict)"(reference=w734) -> (reference out=w737:refnum<vi>, error out=w738:errorcluster, "Value"=w739:i32)  [unwired: 1 in]
                    n503 = Increment(x=w739) -> (x+1=w740:i32)
                    n504 = property class="DigNum (strict)"(reference=w737, error in=w738, "Value"=w740) -> (reference out=w736:refnum<vi>, error out=w735:errorcluster)
                    n505 = Close Reference(reference=w736, error in (no error)=w735) -> ()  [unwired: 1 out]
                  }
                  frame #1 {
                    n506 = Unbundle By Name(w742) -> ("Traction reciepe.SRR INDEX [ STRIBECK]"=w743:refnum<vi>)
                    n507 = Unbundle By Name(w742) -> ("Traction reciepe.Stribeck Size"=w748:refnum<vi>)
                    n508 = property class="DigNum (strict)"(reference=w748) -> (reference out=w746:refnum<vi>, error out=w747:errorcluster, "Value"=w750:i32)  [unwired: 1 in]
                    n509 = property class="DigNum (strict)"(reference=w743) -> (reference out=w745:refnum<vi>, error out=w744:errorcluster, "Value"=w749:i32)  [unwired: 1 in]
                    n510 = Close Reference(reference=w746, error in (no error)=w747) -> ()  [unwired: 1 out]
                    n511 = Close Reference(reference=w745, error in (no error)=w744) -> ()  [unwired: 1 out]
                    n512 = Greater Or Equal?(x=w749, y=w750) -> (x >= y?=w741:bool)
                    n513 = case shown="True" w741 {
                      tunnel: w742 -> [_ w757]
                      frame False {
                      }
                      frame True {
                        n514 = Unbundle By Name(w757) -> ("Traction reciepe.SRR INDEX [ STRIBECK]"=w758:refnum<vi>)
                        n515 = Unbundle By Name(w757) -> ("Traction reciepe.Start Index Type"=w759:refnum<vi>)
                        n516 = property class="DigNum (strict)"(reference=w759) -> (reference out=w762:refnum<vi>, error out=w763:errorcluster, "Value"=w764:i32)  [unwired: 1 in]
                        n517 = property class="DigNum (strict)"(reference=w758, "Value"=0 ("SRR INDEX [ STRIBECK]")) -> (reference out=w755:refnum<vi>, error out=w756:errorcluster)  [unwired: 1 in]
                        n518 = Increment(x=w764) -> (x+1=w765:i32)
                        n519 = Close Reference(reference=w755, error in (no error)=w756) -> ()  [unwired: 1 out]
                        n520 = property class="DigNum (strict)"(reference=w762, error in=w763, "Value"=w765) -> (reference out=w761:refnum<vi>, error out=w760:errorcluster)
                        n521 = Close Reference(reference=w761, error in (no error)=w760) -> ()  [unwired: 1 out]
                      }
                    }
                    n522 = Select(t=Traction_Receipe_Enum."START" ("Enum - Menu"), s=w741, f=Traction_Receipe_Enum."STRIBECK") -> (s? t:f=w752:T2)
                  }
                  frame #2 {
                    n523 = Unbundle By Name(w773) -> ("Traction reciepe.Start Index Type"=w774:refnum<vi>)
                    n524 = property class="DigNum (strict)"(reference=w774) -> (reference out=w776:refnum<vi>, error out=w775:errorcluster, "Value"=w772:i32)  [unwired: 1 in]
                    n525 = Index Array(array=w777, index (row)=w772) -> (element=w783:string[])  [unwired: 1 in]
                    n526 = Close Reference(reference=w776, error in (no error)=w775) -> ()  [unwired: 1 out]
                    n527 = Index Array(array=w783, index=1) -> (element=w771:string)
                    n528 = Equal?(x=w771, y="\"TRACTION\"") -> (x = y?=w768:bool)
                    n529 = call <vilib>:"Trim Whitespace.vi"("string"=w771) -> ("trimmed string"=w769:string)  [unwired: 1 in]
                    n530 = Equal?(x=w769, y="") -> (x = y?=w767:bool)
                    n531 = Or(x=w768, y=w767) -> (x .or. y?=w766:bool)
                    n532 = Select(t=Traction_Receipe_Enum."UNLOAD", s=w766, f=w779) -> (s? t:f=w780:T2)
                  }
                }
                n533 = property class="MCListbox (strict)"(reference=w715) -> (reference out=w713:refnum<vi>, error out=w714:errorcluster, "ItemNames"=w712:string[][])  [unwired: 1 in]
                n534 = property class="Bool (strict)"(reference=w729) -> (reference out=w731:refnum<vi>, error out=w730:errorcluster, "Value"=w728:bool)  [unwired: 1 in]
                n535 = property class="Bool (strict)"(reference=w726) -> (reference out=w724:refnum<vi>, error out=w725:errorcluster, "Value"=w727:bool)  [unwired: 1 in]
                n536 = Close Reference(reference=w731, error in (no error)=w730) -> ()  [unwired: 1 out]
                n537 = Close Reference(reference=w724, error in (no error)=w725) -> ()  [unwired: 1 out]
                n538 = Close Reference(reference=w713, error in (no error)=w714) -> ()  [unwired: 1 out]
                n539 = Equal?(x=w728, y=TRUE) -> (x = y?=w723:bool)
                n540 = Equal?(x=w727, y=FALSE) -> (x = y?=w722:bool)
                n541 = And(x=w723, y=w722) -> (x .and. y?=w719:bool)
                n542 = Select(t=Traction_Receipe_Enum."UNLOAD", s=w719, f=w717) -> (s? t:f=w716:T2)
              }
              frame "UNLOAD" {
                (unwired) FALSE ("Value")
                n543 = call "Test Stop Traction.vi"("Data Cluster"=w784) -> ()  [unwired: 10 in, 1 out]
                n544 = Unbundle By Name(w784) -> ("Traction reciepe.Start Index Type"=w791:refnum<vi>)
                n545 = Unbundle By Name(w784) -> ("Main Screen.Start Test Temp"=w820:refnum<vi>)
                n546 = Unbundle By Name(w784) -> ("Traction reciepe.Test Array Size"=w795:refnum<vi>)
                n547 = Unbundle By Name(w784) -> ("Main Screen.Load En"=w806:refnum<vi>)
                n548 = Unbundle By Name(w784) -> ("Main Screen.STOP"=w823:refnum<vi>)
                n549 = Unbundle By Name(w784) -> ("Main Screen.zNL 2"=w801:refnum<vi>)
                n550 = Unbundle By Name(w784) -> ("Traction reciepe.Traction Receipe Update Details"=w787:refnum<vi>)
                n551 = property on="Property Node" class="DigNum (strict)"(reference=w791) -> (reference out=w790:refnum<vi>, error out=w792:errorcluster, "Value"=w789:i32)  [unwired: 1 in]
                n552 = property class="DigNum (strict)"(reference=w795) -> (reference out=w794:refnum<vi>, error out=w796:errorcluster, "Value"=w793:i32)  [unwired: 1 in]
                n553 = property on="Property Node" class="Bool (strict)"(reference=w806, "Value"=FALSE) -> (reference out=w804:refnum<vi>, error out=w805:errorcluster)  [unwired: 1 in]
                n554 = property class="Bool (strict)"(reference=w823) -> (reference out=w825:refnum<vi>, error out=w824:errorcluster, "Value"=w822:bool)  [unwired: 1 in]
                n555 = property class="Bool (strict)"(reference=w820) -> (reference out=w818:refnum<vi>, error out=w819:errorcluster, "Value"=w821:bool)  [unwired: 1 in]
                n556 = property class="Bool (strict)"(reference=w787, "Value"=FALSE) -> (reference out=w786:refnum<vi>, error out=w788:errorcluster)  [unwired: 1 in]
                n557 = Close Reference(reference=w825, error in (no error)=w824) -> ()  [unwired: 1 out]
                n558 = Close Reference(reference=w818, error in (no error)=w819) -> ()  [unwired: 1 out]
                n559 = Close Reference(reference=w790, error in (no error)=w792) -> ()  [unwired: 1 out]
                n560 = Close Reference(reference=w794, error in (no error)=w796) -> ()  [unwired: 1 out]
                n561 = Close Reference(reference=w786, error in (no error)=w788) -> ()  [unwired: 1 out]
                n562 = Close Reference(reference=w804, error in (no error)=w805) -> (error out=w800:errorcluster)
                n563 = Decrement(x=w793) -> (x-1=w826:i32)
                n564 = Equal?(x=w822, y=TRUE) -> (x = y?=w817:bool)
                n565 = Equal?(x=w821, y=FALSE) -> (x = y?=w816:bool)
                n566 = property on="Property Node" class="Bool (strict)"(reference=w801, error in=w800, "DisabledEnum"=T4."Enabled" ("Disabled")) -> (reference out=w803:refnum<vi>, error out=w802:errorcluster)
                n567 = Greater Or Equal?(x=w789, y=w826) -> (x >= y?=w829:bool)
                n568 = And(x=w817, y=w816) -> (x .and. y?=w813:bool)
                n569 = Select(t=Traction_Receipe_Enum."CLOSE" ("Enum - Menu"), s=w829, f=Traction_Receipe_Enum."START" ("Enum - Menu")) -> (s? t:f=w811:T2)
                n570 = Close Reference(reference=w803, error in (no error)=w802) -> (error out=w797:errorcluster)
                n571 = Select(t=Traction_Receipe_Enum."CLOSE", s=w813, f=w811) -> (s? t:f=w810:T2)
                n572 = call "Reciepe Ball Speed Write.vi"("error in (no error)"=w797, "Set Speed"=0.0, "main ref"=w784) -> ("error out"=w807:errorcluster)  [unwired: 8 in]
                n573 = call "Reciepe Disc Speed Write.vi"("error in (no error)"=w807, "Set Speed"=0.0, "main ref"=w784) -> ()  [unwired: 8 in, 1 out]
              }
              frame "CLOSE" {
                w842 = 0 ("Start Index")
                n574 = call "Test Stop.vi"("Data Cluster"=w832) -> ()  [unwired: 10 in, 1 out]
                n575 = Unbundle By Name(w832) -> ("Traction reciepe.SRR INDEX [ TRACTION]"=w846:refnum<vi>)
                n576 = Unbundle By Name(w832) -> ("Traction reciepe.SRR INDEX [ STRIBECK]"=w843:refnum<vi>)
                n577 = Unbundle By Name(w832) -> ("Main Screen.Start Test Temp"=w835:refnum<vi>)
                n578 = Unbundle By Name(w832) -> ("Traction reciepe.Start Index Type"=w850:refnum<vi>)
                n579 = Unbundle By Name(w832) -> ("Traction reciepe.Traction Receipe Update Details"=w840:refnum<vi>)
                n580 = call "Temperature vi FGV.vi"("Enum"=Temperature_enum."write", "Set Temperature"=0.0, "main ref"=w832) -> ("error out"=→"error out 2":errorcluster)  [unwired: 8 in]
                n581 = property class="Bool (strict)"(reference=w835, "Value"=FALSE) -> (reference out=w834:refnum<vi>, error out=w836:errorcluster)  [unwired: 1 in]
                n582 = property class="DigNum (strict)"(reference=w850, "Value"=w842) -> (reference out=w849:refnum<vi>, error out=w851:errorcluster)  [unwired: 1 in]
                n583 = property class="DigNum (strict)"(reference=w846, "Value"=w842) -> (reference out=w848:refnum<vi>, error out=w847:errorcluster)  [unwired: 1 in]
                n584 = property class="DigNum (strict)"(reference=w843, "Value"=w842) -> (reference out=w845:refnum<vi>, error out=w844:errorcluster)  [unwired: 1 in]
                n585 = Close Reference(reference=w834, error in (no error)=w836) -> ()  [unwired: 1 out]
                n586 = property class="Bool (strict)"(reference=w840, "Value"=FALSE) -> (reference out=w839:refnum<vi>, error out=w841:errorcluster)  [unwired: 1 in]
                n587 = Close Reference(reference=w849, error in (no error)=w851) -> ()  [unwired: 1 out]
                n588 = Close Reference(reference=w848, error in (no error)=w847) -> ()  [unwired: 1 out]
                n589 = Close Reference(reference=w845, error in (no error)=w844) -> ()  [unwired: 1 out]
                n590 = Close Reference(reference=w839, error in (no error)=w841) -> ()  [unwired: 1 out]
              }
            }
            n591 = property class="Enum (strict)"(reference=w33, "Value"=w30) -> (reference out=w31:refnum<vi>, error out=w34:errorcluster)  [unwired: 1 in]
            n592 = Close Reference(reference=w31, error in (no error)=w34) -> ()  [unwired: 1 out]
          }
        }
      }
    }
    frame Error {
    }
  }
